vi "WS1050 36 DUT CV Curve Ver1.1.vi"() -> ()   [LabVIEW 2012]
uses:
  All Driver/Keithley/2012_Keithley 24XX/Keithley 24XX.lvlib
  WS_VCAP Driver 029/Source/WSVCAP Shell/Type Defs/WSVCAP SHL I2C DUT Mask Mode Enum.ctl
panel:
  out "VISA resource name out":refnum<visa-resource-name>="GPIB0::3::INSTR"
  out "error out 2":errorcluster={"status"=TRUE, "code"=-63192, "source"="niLvFpga_Open_PXI-7813R.vi"}
  in  "Reg1_Bit Cntrl":string[](array[string])=["01", "02", "04", "08", "10", "20", "40", "80", "03", "06", "0C", "D8", "33", "66", "CC", "07", "0E", "1C", "38", "70", "E0", "0F", "1E", "3C", "78", "F0", "1F", "3E", "7C", "F8", "3F", "7E", "FC", "7F", "FE", "FD", "FB", "F7", "EF", "DF", "BF", "7F", "FC", "F9", "F3", "E7", "CF", "9F", "3F", "F8", "F1", "E3", "C7", "8F", "1F", "F0", "E1", "C3", "87", "0F", "E0", "C1", "83", "07", "C0", "81", "03", "AA", "55", "00"]
  out "date string":string="5/19/2014"
  out "PS1 Out":refnum<visa-resource-name>
  out "Ke2000 Out":refnum<visa-resource-name>="GPIB0::9::INSTR"
  in  "Tab Control":T1(tab)
  in  "Board#":string="BRD5"
  in  "Serial Number":string[][](table)=[["DUT", "SN"], ["DUT1", "1"], ["DUT2", "2"], ["DUT3", "3"], ["DUT4", "4"], ["DUT5", "5"], ["DUT6", "6"], ["DUT7", "7"], ["DUT8", "8"], ["DUT9", "9"], ["DUT10", "10"], ["DUT11", "11"], ["DUT12", "12"], ["DUT13", "13"], ["DUT14", "14"], ["DUT15", "15"], ["DUT16", "16"], ["DUT17", "17"], ["DUT18", "18"], ["DUT19", "19"], ["DUT20", "20"], ["DUT21", "21"], ["DUT22", "22"], ["DUT23", "23"], ["DUT24", "24"], ["DUT25", "25"], ["DUT26", "26"], ["DUT27", "27"], ["DUT28", "28"], ["DUT29", "29"], ["DUT30", "30"], ["DUT31", "31"], ["DUT32", "32"], ["DUT33", "33"], ["DUT34", "34"], ["DUT35", "35"], ["DUT36", "36"]]
  in  "Wafer#":string="T7-EB"
  in  "File Name":string="CYC_WS1050_T7_EB_65C_40V_25DC_EMPTY_BRD5_141017_1"
  in  "TMN DC\\CAP Data Log File Path":path=path "C:/WS1050 36 DUT Data"
  in  "Test Program":string="WS1050 36 DUT CV Curve Ver1.1"
  out "Current Date":string="8/28/2014"
  out "Current Time":string="0950"
  in  "Start Date":string="10/21/2014"
  in  "Start Time":string="1542"
  in  "Comment":string="CYC65C40V"
  in  "OK Button":bool
  in  "Calibration":bool
  in  "Verify CP":bool
  in  "CP Setting":i32(ring) items=["CP OFF", "CP ON", "CP 35V", "CP 40V", "DVA ON", "DVA OFF", "REG1 ON", "REG1 OFF", "REG2 ON", "REG2 OFF", "REG3 ON", "REG3 OFF"]
  in  "Stop Calibration":bool
  in  "Set VDD":dbl=3.3 format="%.3g"
  in  "Clock Rate (Hz)":dbl=1000000.0 caption="Meas Speed" format="%.1p Hz"
  out "AR  Measurent(Hz)":dbl
  in  "PS1 Source":refnum<visa-resource-name>="GPIB0::5::INSTR"
  in  "Ke2000":refnum<visa-resource-name>="GPIB0::9::INSTR"
  in  "CP to HD/Cycle":i32(ring)=1 items=["CP HDC 35V", "CP HDC 40.25V", "CP HDC 27.5V", "CP HDC 30.5V", "CP HDC 44V"]
  out "Simulate FPGA":bool
  out "Online":bool
  in  "Ke2400":refnum<visa-resource-name>="GPIB0::3::INSTR"
  in  "Initialize AD7747":bool
  in  "DUT Mask Mode":T2=enum."All"
  in  "RFFE Slave Address":u8=7 caption="Slave Address" format="0x%02x"
  out "Activity Log":string="05/19/2014 -- 12:24:35.853::WSVCAP::APP::Application Started\n05/19/2014 -- 12:24:37.606::WSVCAP::WSVCAP SHL::WR I2C-REG:0x0A;MASK:0xFFFFFFFFFFFF;C1 DATA:22:22:22:22:22:22:22:22:22:22:22:22:22:22:22:22;C2 DATA:22:22:22:22:22:22:22:22:22:22:22:22:22:22:22:22;C3 DATA:22:22:22:22:22:22:22:22:22:22:22:22:22:22:22:22\r\n05/19/2014 -- 12:24:37.773::WSVCAP::WSVCAP SHL::WR I2C-ST:0,0,4,1\r\n05/19/2014 -- 12:24:37.903::WSVCAP::WSVCAP SHL::RD I2C-BYTES:4;ADD:0x00;MASK:0xFFFFFFFFFFFF\r\n05/19/2014 -- 12:24:38.045::WSVCAP::WSVCAP SHL::RD I2C:C1 DATA:2:2:2:2:2:2:2:2:2:2:2:2:2:2:2:2|A7:A9:AA:82:82:7F:82:81:82:81:83:82:81:82:82:81|46:36:BB:88:44:A3:E9:2B:32:20:ED:25:BB:3D:68:B|2C:6A:EB:A7:22:56:FE:CC:36:82:D7:B0:3B:48:F9:CC;C2 DATA:2:2:2:2:2:2:2:2:2:2:2:2:2:2:2:2|94:94:94:80:80:80:80:80:81:7E:7E:81:80:7E:80:80|47:33:15:82:62:B:E8:1C:D7:C3:7D:41:7C:B7:4C:2A|C4:B4:AE:8:1E:D1:4E:37:11:C0:6F:63:42:9D:63:B5;C3 DATA:2:2:2:2:2:2:2:2:2:2:2:2:2:2:2:2|95:95:95:81:81:7E:81:80:84:7D:80:83:81:7E:7F:80|AB:C4:14:B5:7B:52:DF:C9:79:5D:5F:30:99:31:1E:F4|6E:5C:F7:A8:C3:EB:7B:EF:33:92:89:77:4D:67:75:DD;STATUS:0:0:4:0\r\n05/19/2014 -- 12:24:38.046::WSVCAP::WSVCAP SHL::WR I2C-REG:0x0A;MASK:0xFFFFFFFFFFFF;C1 DATA:22:22:22:22:22:22:22:22:22:22:22:22:22:22:22:22;C2 DATA:22:22:22:22:22:22:22:22:22:22:22:22:22:22:22:22;C3 DATA:22:22:22:22:22:22:22:22:22:22:22:22:22:22:22:22\r\n05/19/2014 -- 12:24:38.089::WSVCAP::WSVCAP SHL::WR I2C-ST:0,0,4,1\r\n05/19/2014 -- 12:24:38.219::WSVCAP::WSVCAP SHL::RD I2C-BYTES:4;ADD:0x00;MASK:0xFFFFFFFFFFFF\r\n05/19/2014 -- 12:24:38.362::WSVCAP::WSVCAP SHL::RD I2C:C1 DATA:2:2:2:2:2:2:2:2:2:2:2:2:2:2:2:2|A7:AB:AA:82:82:82:83:83:82:82:82:82:7F:82:82:81|4B:32:96:83:3E:61:43:17:25:62:AB:4D:A2:40:2E:5|3C:76:2B:B4:EE:E4:A9:1A:AA:A:26:C7:21:2E:87:5B;C2 DATA:2:2:2:2:2:2:2:2:2:2:2:2:2:2:2:2|94:94:94:80:80:80:80:80:80:7F:80:81:80:80:7F:80|4A:32:19:7D:19:6C:79:46:61:7F:4B:B8:A5:30:F3:14|B4:70:A:8C:9C:DC:43:FA:1E:A:C6:21:A:A9:13:F3;C3 DATA:2:2:2:2:2:2:2:2:2:2:2:2:2:2:2:2|95:97:94:81:80:81:82:81:80:7E:81:84:7F:81:80:80|B2:32:D0:A7:9E:4C:AB:D4:EE:D9:F0:82:B7:91:7:FF|C1:91:B6:3D:D8:E:1B:4F:9F:6A:F1:6C:E7:3F:7:BA;STATUS:0:0:4:0\r\n05/19/2014 -- 12:24:38.364::WSVCAP::WSVCAP SHL::WR I2C-REG:0x0A;MASK:0xFFFFFFFFFFFF;C1 DATA:22:22:22:22:22:22:22:22:22:22:22:22:22:22:22:22;C2 DATA:22:22:22:22:22:22:22:22:22:22:22:22:22:22:22:22;C3 DATA:22:22:22:22:22:22:22:22:22:22:22:22:22:22:22:22\r\n05/19/2014 -- 12:24:38.406::WSVCAP::WSVCAP SHL::WR I2C-ST:0,0,4,1\r\n05/19/2014 -- 12:24:38.536::WSVCAP::WSVCAP SHL::RD I2C-BYTES:4;ADD:0x00;MASK:0xFFFFFFFFFFFF\r\n05/19/2014 -- 12:24:38.678::WSVCAP::WSVCAP SHL::RD I2C:C1 DATA:2:2:2:2:2:2:2:2:2:2:2:2:2:2:2:2|A7:A9:AB:82:82:81:82:82:82:82:82:82:82:82:82:81|46:71:4C:87:43:3D:7F:FC:25:4F:8E:54:97:3E:60:8C|AA:F4:1F:B5:CE:43:1F:36:9:87:9C:78:86:5:B6:8E;C2 DATA:2:2:2:2:2:2:2:2:2:2:2:2:2:2:2:2|94:94:94:80:7F:7F:80:80:80:80:80:81:80:80:80:80|49:36:18:7D:6E:C5:E4:3C:81:2E:41:D3:75:71:E3:72|E8:D3:E6:D1:E0:48:AE:D4:54:D:E8:8E:B4:41:68:4;C3 DATA:2:2:2:2:2:2:2:2:2:2:2:2:2:2:2:2|95:95:95:81:7F:7F:81:81:81:81:81:84:81:81:82:81|B3:F5:90:AB:82:69:7B:93:D0:77:E8:D5:E8:8C:84:E8|B9:AC:EE:2B:B6:71:8F:4A:74:31:56:BB:8A:B7:A0:C8;STATUS:0:0:4:0\r\n05/19/2014 -- 12:24:38.681::WSVCAP::WSVCAP SHL::WR I2C-REG:0x0A;MASK:0xFFFFFFFFFFFF;C1 DATA:22:22:22:22:22:22:22:22:22:22:22:22:22:22:22:22;C2 DATA:22:22:22:22:22:22:22:22:22:22:22:22:22:22:22:22;C3 DATA:22:22:22:22:22:22:22:22:22:22:22:22:22:22:22:22\r\n05/19/2014 -- 12:24:38.723::WSVCAP::WSVCAP SHL::WR I2C-ST:0,0,4,1\r\n05/19/2014 -- 12:24:38.854::WSVCAP::WSVCAP SHL::RD I2C-BYTES:4;ADD:0x00;MASK:0xFFFFFFFFFFFF\r\n05/19/2014 -- 12:24:38.996::WSVCAP::WSVCAP SHL::RD I2C:C1 DATA:2:2:2:2:2:2:2:2:2:2:2:2:2:2:2:2|A7:A9:AA:82:82:7F:83:81:82:81:84:82:7F:82:7F:82|43:FB:E:7F:3C:AD:35:35:26:A2:6C:21:4B:3D:8:6|63:9A:E1:F3:95:32:91:42:90:3C:78:1F:5C:D7:5F:D8;C2 DATA:2:2:2:2:2:2:2:2:2:2:2:2:2:2:2:2|94:94:94:80:80:80:80:80:81:80:7E:81:80:7E:7F:80|48:36:18:7F:5E:3D:69:83:DE:AE:A1:9E:31:AE:BB:96|15:A0:44:17:13:FD:CC:C8:6D:B2:EF:A7:C:C7:3B:F;C3 DATA:2:2:2:2:2:2:2:2:2:2:2:2:2:2:2:2|95:96:94:81:81:7E:82:80:84:80:80:84:7F:7E:7D:82|AD:3B:6D:A9:7C:57:9D:F5:7A:96:23:5C:36:2D:ED:5A|CD:46:DB:3B:C7:BD:70:60:33:B8:B:F7:63:A:51:4D;STATUS:0:0:4:0\r\n05/19/2014 -- 12:24:38.998::WSVCAP::WSVCAP SHL::WR I2C-REG:0x0A;MASK:0xFFFFFFFFFFFF;C1 DATA:22:22:22:22:22:22:22:22:22:22:22:22:22:22:22:22;C2 DATA:22:22:22:22:22:22:22:22:22:22:22:22:22:22:22:22;C3 DATA:22:22:22:22:22:22:22:22:22:22:22:22:22:22:22:22\r\n05/19/2014 -- 12:24:39.040::WSVCAP::WSVCAP SHL::WR I2C-ST:0,0,4,1\r\n05/19/2014 -- 12:24:39.170::WSVCAP::WSVCAP SHL::RD I2C-BYTES:4;ADD:0x00;MASK:0xFFFFFFFFFFFF\r\n05/19/2014 -- 12:24:39.311::WSVCAP::WSVCAP SHL::RD I2C:C1 DATA:2:2:2:2:2:2:2:2:2:2:2:2:2:2:2:2|A7:AA:AB:82:82:81:82:81:82:81:82:82:82:82:7F:82|44:F1:90:87:45:44:C8:2C:2C:F1:FC:1B:94:3B:3C:75|4A:49:95:19:99:73:64:3:23:24:F3:A2:5E:7F:C4:B6;C2 DATA:2:2:2:2:2:2:2:2:2:2:2:2:2:2:2:2|94:94:94:80:80:80:80:7F:80:80:7E:80:80:7E:7F:80|4C:36:17:7D:A8:9F:DE:C7:53:6D:8A:F4:41:A5:C6:E0|90:2E:24:C:D9:22:E4:76:3B:40:1D:53:33:B1:3E:4D;C3 DATA:2:2:2:2:2:2:2:2:2:2:2:2:2:2:2:2|95:97:95:81:81:7F:81:80:80:81:7F:82:81:7E:7D:82|AE:2B:A7:AB:CC:CD:A4:38:FD:17:80:F2:92:2D:45:C4|76:E5:D:B9:AD:B5:BA:8D:28:32:9E:42:B7:20:4A:D9;STATUS:0:0:4:0\r\n05/19/2014 -- 12:24:39.313::WSVCAP::WSVCAP SHL::WR I2C-REG:0x0A;MASK:0xFFFFFFFFFFFF;C1 DATA:22:22:22:22:22:22:22:22:22:22:22:22:22:22:22:22;C2 DATA:22:22:22:22:22:22:22:22:22:22:22:22:22:22:22:22;C3 DATA:22:22:22:22:22:22:22:22:22:22:22:22:22:22:22:22\r\n05/19/2014 -- 12:24:39.355::WSVCAP::WSVCAP SHL::WR I2C-ST:0,0,4,1\r\n05/19/2014 -- 12:24:39.486::WSVCAP::WSVCAP SHL::RD I2C-BYTES:4;ADD:0x00;MASK:0xFFFFFFFFFFFF\r\n05/19/2014 -- 12:24:39.628::WSVCAP::WSVCAP SHL::RD I2C:C1 DATA:2:2:2:2:2:2:2:2:2:2:2:2:2:2:2:2|A7:A9:AA:82:82:82:83:82:82:82:82:82:7F:82:7F:82|47:18:E4:87:3E:E7:6:65:25:92:37:38:A8:3E:89:85|7C:A7:7:2B:A3:7A:EC:EF:89:ED:F4:D3:D8:BC:3A:F5;C2 DATA:2:2:2:2:2:2:2:2:2:2:2:2:2:2:2:2|94:94:94:80:7F:80:80:7F:81:80:7E:80:80:80:81:80|49:37:17:80:76:25:6A:F8:DF:55:97:4D:B8:5B:2B:B1|13:E3:9A:3E:1A:2D:4F:B6:DB:E9:61:FA:8B:D6:9:CC;C3 DATA:2:2:2:2:2:2:2:2:2:2:2:2:2:2:2:2|95:95:95:81:7F:80:82:81:84:80:7F:81:80:81:7F:82|AF:93:3B:AF:5B:11:82:E4:7E:C3:2D:72:9:96:D9:A|DB:96:F2:10:5F:64:9A:C6:98:12:27:7D:10:D3:20:D9;STATUS:0:0:4:0\r\n05/19/2014 -- 12:24:40.132::WSVCAP::WSVCAP SHL::CLOSE\r\n"
  in  "C1 Cap DAC":u8=128 caption="B Data In" format="0x%02x"
  in  "C2 Cap DAC":u8=128 caption="B Data In" format="0x%02x"
  in  "C3 Cap DAC":u8=128 caption="B Data In" format="0x%02x"
  out "IDD Brd(uA)":string
  in  "Control Panel":T3={"Verify Socket"=FALSE, "HD/CYC"=FALSE, "E-CAL"=FALSE, "DVA"=FALSE, "VPI"=TRUE, "VSA"=FALSE, "HS"=FALSE}
  out "Verify Socket":bool
  out "HD/CYC":bool
  out "E-CAL":bool
  out "DVA":bool
  out "VPI":bool
  out "VSA":bool
  out "HS":bool
  in  "Lot#":string="WS1050"
  out "AD7747 Values":string[][](table)
  in  "Freq(Hz)":string="NA"
  in  "Reset P/S":bool
  in  "Test Sequences":i32(ring) items=["C1_C2_C3", "C2_C1_C3", "C3_C2_C1"]
  in  "WS1050/51":bool=TRUE
  in  "CP with DVA ON":i32(ring) items=["CP HDC 35V", "CP HDC 40.25V", "CP HDC 27.5V", "CP HDC 30.5V", "CP HDC 44V"]
  in  "CP Sweep":bool=TRUE
  in  "Serialize":bool
  in  "Start No":i32=1
  in  "VPI Name":string[](array[string])=["All Drivers ON"]
  in  "VPI_Cmd":string[](array[string])=["3B"]
  in  "Temperature":string="25C"
  out "40V_1":string[][](table)
  out "NOM IDD OFF(uA)":string
  out "40V_2":string[][](table)
  out "40V_3":string[][](table)
  out "Previous Time":string="12:20:26 PM"
  out "STATUS":string="Idle...."
  out "Total Delta C2(pF)":string[](array[string])
  out "Total Delta C1(pF)":string[](array[string])
  out "Total Delta C3(pF)":string[](array[string])
  out "RB Reg for HD/Cycle":string[](array[string])
  out "VPI C2":string[][](table)
  out "VPI C3":string[][](table)
  out "NOM IDD ON (uA)":string
  out "IDD_HD/CYC (uA)":string="164.601255E+0"
  in  "stop":bool
  out "IDD Stdby(uA)":string="2.606990E+0"
  out "VPI C1":string[][](table)
  in  "TTF Completed":i32=60
  out "Loop Completed":i32
  out "VSA_V1":string[][](table)
  out "VSA_V2":string[][](table)
  out "VSA_V3":string[][](table)
  in  "VSA Voltage(V)":dbl[](array[numeric])=[-27.0, 0.0, 27.0]
  in  "X Repeat":i32=100
  out "% Delta C_T0":string[][](array[string])
  out "% Delta C":string[][](array[string])
  out "EFuse RB T0":string[](array[string])
  out "Current EFuse Read back":string[](array[string])
  out "EFuse Readback Status":bool[](array[boolean])
  in  "DeltaC Target Setting(pF)":dbl=7.375
  out "error out":errorcluster
  in  "error in (no error)":errorcluster
  in  "Bank 2":i32(ring)=1 items=["C1", "C2", "C3", "D_C1", "D_C2", "D_C3"]
  out "DeltaC Change_1":dbl[][](graph) caption="(Y) Multi Plot 2"
  out "DeltaC Change_2":dbl[][](graph) caption="(Y) Multi Plot 2"
  out "DeltaC Change_3":dbl[][](graph) caption="(Y) Multi Plot 2"
  in  "Debug":bool
  in  "No of Rows\nFrom Spread Sheet":i32
  in  "Plot Delta Cmin":bool=TRUE
  in  "Plot":T4(ring)
  in  "Bank 1":i32(ring) items=["C1", "C2", "C3", "D_C1", "D_C2", "D_C3"]
  in  "Bank 3":i32(ring)=2 items=["C1", "C2", "C3", "D_C1", "D_C2", "D_C3"]
  in  "Col C1":i32=5
  in  "Col C2":i32=6
  in  "Col C3":i32=7
  # "Company:  WiSpry Inc\n20 Fairbanks Ste 198 Irvine CA 92618\n\nAuthor:  Andy V Tran\nCreated:  01/07/2015\nLabVIEW 2012 Pro\nTest Program:  WS1050 36 DUT CV Curve ver1.0\nFPGA: WS_VCAP Driver 029"
  # "Note for HD Duty Cycle:\n\n1.  Set HD/Cycle to Completed = 4320 minutes = 72 hours \n(T0 24hrs HD, T2 48hrs HD_Duty Cycle);  Default Setting\n2.  Set Time to Start HD Duty Cycle = 1440 = 24 hours\n3.  Set Time All ON = 120s = 2 minutes\n4.  Set Time All OFF = 120s = 2 minutes\n5.  No of Loops to RP = 3600s/(Time ALL ON(s) + Time ALL + OFF(s))\n6.  X Repeat = X runs\n7.  Set TTF Completed = Repeat X item1 to Stop.\n8.  Stop Test, set TTF Completed = Total Time Completed."
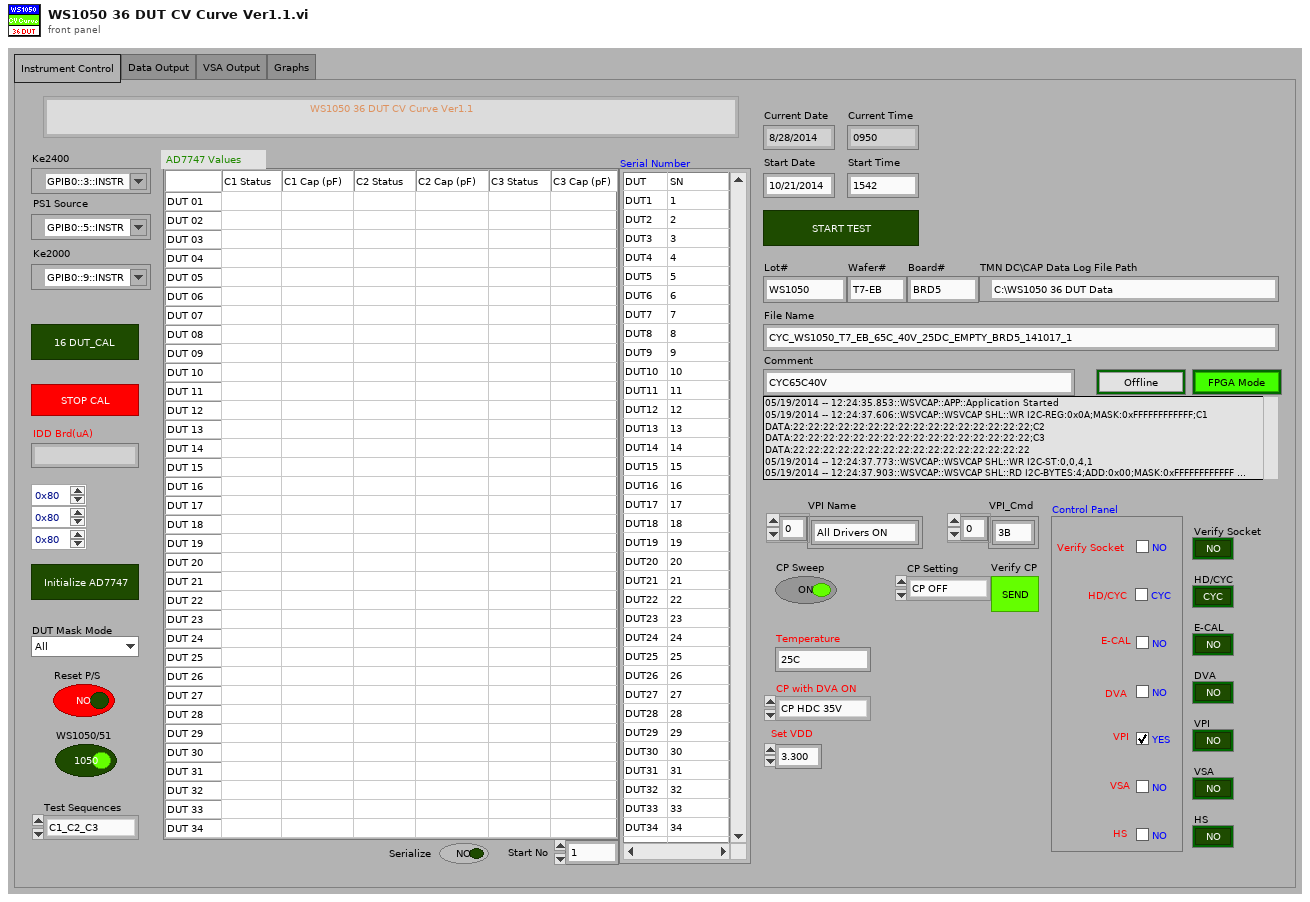
[diagram p1: front panel]
types:
  T1 = enum32{"Instrument Control", "Data Output", "VSA Output", "Graphs"}
  T2 = typedef "WSVCAP SHL I2C DUT Mask Mode Enum.ctl" = enum16{"Custom", "C1", "C2", "C3", "All"}
  T3 = cluster{"Verify Socket":bool, "HD/CYC":bool, "E-CAL":bool, "DVA":bool, "VPI":bool, "VSA":bool, "HS":bool}
  T4 = enum16{"ALL DUTs", "DUT 01", "DUT 02", "DUT 03", "DUT 04", "DUT 05", "DUT 06", "DUT 07", "DUT 08", "DUT 09", "DUT 10", "DUT 11", "DUT 12", "DUT 13", "DUT 14", "DUT 15", "DUT 16", "DUT 17", "DUT 18", "DUT 19", "DUT 20", "DUT 21", "DUT 22", "DUT 23", "DUT 24", "DUT 25", "DUT 26", "DUT 27", "DUT 28", "DUT 29", "DUT 30", "DUT 31", "DUT 32", "DUT 33", "DUT 34", "DUT 35", "DUT 36"}
  T5 = typedef "WSVCAP SHL Core System Cluster.ctl" = cluster{"Settings":T6, "FPGA Resource":tag, "Online":bool, "I2C Wait Ticks":u32, "SPI Wait Ticks":u32, "RFFE Wait Ticks":u32}
  T6 = typedef "WSVCAP SHL I2C Settings Cluster.ctl" = cluster{"FPGA Resource Name":string, "I2C Slave Address":u8, "I2C Clock Rate (Hz)":dbl, "SPI Clock Rate (Hz)":dbl, "RFFE Slave Address":u8, "RFFE Clock Rate (Hz)":dbl, "Simulate FPGA":bool, "C1 Cap DAC Default":u8, "C2 Cap DAC Default":u8, "C3 Cap DAC Default":u8}
  T7 = enum16{"Idle...", "Voltage 1", "Voltage 2", "Voltage 3"}[]
  T8 = cluster{"Test Program ":string, "Comment":string, "Data Out":string, "Data Out":string, "Data Out":string, string, "Data Out":string, "Data Out":string, "Data Out":string, "Freq(Hz)":string, "Board#":string}
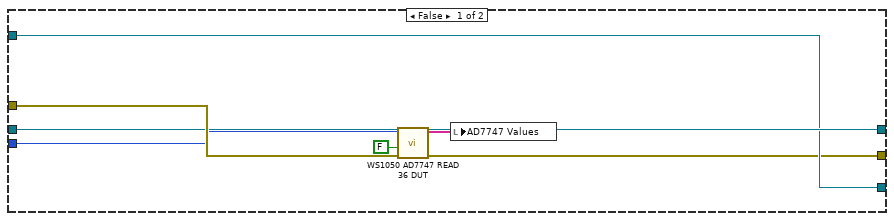
[diagram p9: hidden frame]
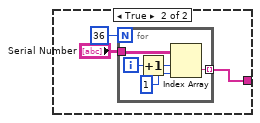
[diagram p10: hidden frame]
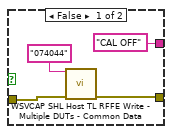
[diagram p11: hidden frame]
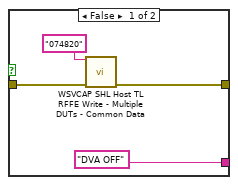
[diagram p12: hidden frame]
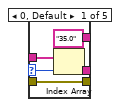
[diagram p13: hidden frame]
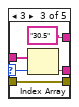
[diagram p14: hidden frame]
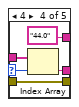
[diagram p15: hidden frame]
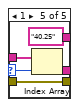
[diagram p16: hidden frame]
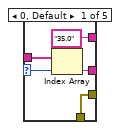
[diagram p17: hidden frame]
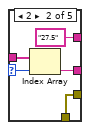
[diagram p18: hidden frame]
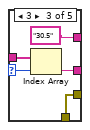
[diagram p19: hidden frame]
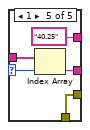
[diagram p20: hidden frame]
diagram:
  w18 = TRUE
  w24 = u16 0 items=["Off", "Moving Filter", "Repeating Filter"] ("Digital Filter (0: Off)")
  w25 = u16 7 items=["3.5 Digits"=4, "4.5 Digits"=5, "5.5 Digits"=6, "6.5 Digits"=7] ("Resolution (7: 6.5 digits)")
  n1 = case shown="True" w18 {
    tunnel: "error in (no error)" -> [w31 w32]
    tunnel: [w31 w39] -> w5
    frame False {
    }
    frame True {
      n2 = call "WSVCAP SHL Host TL Initialize.vi"("error in"=w32) -> ("error out"=w33:errorcluster)  [unwired: 13 in, 1 out]
      n3 = control-ref of="Activity Log"() -> (w35:refnum<vi>)
      n4 = call "ACT LG Activity Log Core.vi"("Display Ref"=w35, "Source"="WSVCAP", "Error In (no error)"=w33) -> ("Error Out"=w34:errorcluster)  [unwired: 11 in, 1 out]
      n5 = call "WSVCAP SHL Host TL Status Manager.vi"("error in"=w34) -> ("System Out"=w40:T5, "error out"=w39:errorcluster)  [unwired: 13 in]
      n6 = Unbundle By Name(w40) -> ("Online"=→"Online":bool, "Settings.Simulate FPGA"=→"Simulate FPGA":bool)
    }
  }
  n7 = case shown="True" TRUE {
    tunnel: w5 -> [w41 w46]
    tunnel: [w42 w45] -> w15
    tunnel: [w41 w44] -> w9
    tunnel: "Ke2400" -> [w42 w43]
    frame False {
    }
    frame True {
      n8 = VISA Write(VISA resource name=w43, write buffer="SOUR:FUNC VOLT;VOLT:MODE FIX;RANG 100;LEV 0.0;:SENS:FUNC \"CURR\";CURR:PROT 60E-3;RANG 100E-3;:OUTP ON", error in (no error)=w46) -> (VISA resource name out=w45:refnum<visa-resource-name>, error out=w44:errorcluster)  [unwired: 1 out]
    }
  }
  n9 = case shown="True" "Reset P/S" {
    tunnel: "PS1 Source" -> [w48 w55]
    tunnel: [w48 w53] -> w29
    tunnel: w5 -> [w49 w51]
    tunnel: [w49 w50] -> w4
    frame False {
    }
    frame True {
      n10 = call "Agilent 3631A Initialize.vi"("error in (no error)"=w51, "Default"=FALSE ("Reset? (T: Yes)"), "Reset"=TRUE ("ID Query? (T: Yes)"), "VISA resource name"=w55) -> ("error out"=w50:errorcluster, "VISA resource name out"=w53:refnum<visa-resource-name>)  [unwired: 6 in]
    }
  }
  n11 = call "Ke2000 Initialize.vi"("error in (no error)"=w5, "VISA resource name"="Ke2000") -> ("error out"=w26:errorcluster, "VISA resource name out"=w27:refnum<visa-resource-name>)  [unwired: 8 in]
  n12 = call "Ke2000 Configure DC Current.vi"("Resolution (7: 6.5 digits)"=w25, "Digital Filter (0: Off)"=w24, "Auto Range? (T: Auto)"=FALSE, "error in"=w26, "Custom Range (0 A)"=1.0, "VISA resource name"=w27) -> ("error out"=w6:errorcluster, "VISA resource name out"=w22:refnum<visa-resource-name>)  [unwired: 4 in]
  n13 = Merge Errors(w9, w6, w4) -> (w16:errorcluster)
  n14 = while {
    tunnel: w16 -> [w61]
    tunnel: [w64] -> w12
    tunnel: w29 -> [w68]
    tunnel: w22 -> [w69]
    tunnel: [w78] -> w21
    tunnel: [w77] -> w20
    tunnel: w15 -> [w75]
    tunnel: [w74] -> w13
    tunnel: [FALSE ("stop")] -> w7
    i -> [w76]
    stop <- w80 stop-if-true
    n15 = case shown="0" w76 {
      tunnel: w61 -> [w91 w92]
      tunnel: [w90 w92] -> w71
      tunnel: "RFFE Slave Address" -> [w88 _]
      frame 0 {
        w84 = dbl[][] []
        w83 = "" ("uA")
        w85 = string[][] []
        w86 = string[] [] ("EFuse Read back")
        n16 = local write "RB Reg for HD/Cycle"(w86) -> ()
        n17 = local write "Current EFuse Read back"(w86) -> ()
        n18 = local write "EFuse RB T0"(w86) -> ()
        n19 = local write "Total Delta C1(pF)"(w86) -> ()
        n20 = local write "Total Delta C2(pF)"(w86) -> ()
        n21 = local write "Total Delta C3(pF)"(w86) -> ()
        n22 = local write "VPI C2"(w85) -> ()
        n23 = local write "VSA_V3"(w85) -> ()
        n24 = local write "VSA_V1"(w85) -> ()
        n25 = local write "40V_2"(w85) -> ()
        n26 = local write "40V_1"(w85) -> ()
        n27 = local write "NOM IDD OFF(uA)"(w83) -> ()
        n28 = local write "NOM IDD ON (uA)"(w83) -> ()
        n29 = local write "IDD Brd(uA)"(w83) -> ()
        n30 = local write "VSA_V2"(w85) -> ()
        n31 = local write "VPI C1"(w85) -> ()
        n32 = local write "VPI C3"(w85) -> ()
        n33 = local write "% Delta C"(w85) -> ()
        n34 = local write "% Delta C_T0"(w85) -> ()
        n35 = local write "40V_3"(w85) -> ()
        n36 = call "WSVCAP SHL Host TL RFFE Configure.vi"("RFFE Slave Address"=w88, "Clock Rate (Hz)"="Clock Rate (Hz)", "error in"=w91) -> ("Actual Rate (Hz)"=→"AR  Measurent(Hz)":dbl, "error out"=w90:errorcluster)  [unwired: 11 in]
        n37 = local write "DeltaC Change_3"(w84) -> ()
        n38 = local write "DeltaC Change_1"(w84) -> ()
        n39 = local write "DeltaC Change_2"(w84) -> ()
      }
      frame 1, Default {
      }
    }
    n40 = while {
      tunnel: ["stop"] -> w73
      tunnel: w71 -> [w113]
      tunnel: [w105] -> w65
      tunnel: w68 -> [w112]
      tunnel: w69 -> [w107]
      tunnel: [w108] -> w67
      tunnel: [w106] -> w66
      tunnel: [w103] -> w63
      tunnel: [w102] -> w62
      tunnel: [w101] -> w60
      tunnel: [w100] -> w59
      tunnel: [w99] -> w58
      tunnel: [w98] -> w57
      tunnel: [w97] -> w56
      stop <- w120 stop-if-true
      # "Set Date & Time to Start Test"
      n41 = case shown="True" "Initialize AD7747" {
        tunnel: w113 -> [w129 w134]
        tunnel: [w129 w130] -> w96
        tunnel: w112 -> [w128 w132]
        tunnel: [w128 w131] -> w111
        frame False {
        }
        frame True {
          w135 = T7 [enum."Voltage 2", enum."Voltage 3", enum."Voltage 1"] items=["Idle...", "Voltage 1", "Voltage 2", "Voltage 3"]
          n42 = for {
            tunnel: w132 -> [w145]
            tunnel: w135 -> [w143] mode=indexing
            tunnel: [w142] -> w131
            shift-right: [w138] -> w133
            shift-left: w134 -> [w146]
            n43 = local read "Set VDD"() -> (w141:dbl)
            n44 = call "E3631A_Voltage Controller.vi"("VISA resource name"=w145, "I_VDD(A)"=0.5, "Channel Controller"=w143, "Voltage 1"=w141, "Voltage 2"=3.3, "error in (no error)"=w146, "I_3.3V (A)"=0.5) -> ("VISA resource name out"=w142:refnum<visa-resource-name>, "error out"=w137:errorcluster)  [unwired: 7 in]
            n45 = call "Delay T4.vi"("milliseconds to wait"=u32 100, "error in (no error)"=w137) -> ("error out"=w138:errorcluster)  [unwired: 9 in]
          }
          n46 = call "WS1050_AD7747_Init 36DUT.vi"("error in"=w133) -> ("error out"=w130:errorcluster)  [unwired: 10 in]
        }
      }
      n47 = call "Time_stamp.vi"() -> ("date/time string"=w125:string, "date string"=w127:string)  [unwired: 2 in]
      "Current Date" <- w127
      "Current Time" <- w125
      n48 = Equal?(x=w127, y="Start Date") -> (x = y?=w123:bool)
      n49 = Equal?(x=w125, y="Start Time") -> (x = y?=w122:bool)
      n50 = And(x=w123, y=w122) -> (x .and. y?=w119:bool)
      n51 = Compound Arithmetic op=OR(w119, "OK Button", "stop") -> (w120:bool)
      n52 = case shown="True" "Calibration" {
        tunnel: w96 -> [w176 w193]
        tunnel: [w170 w190] -> w94
        tunnel: w111 -> [w175 w189]
        tunnel: "DUT Mask Mode" -> [w174 w185]
        tunnel: [w175 w184] -> w109
        tunnel: w107 -> [w173 w180]
        tunnel: [w173 w177] -> w106
        frame False {
          n53 = call "WS1050 AD7747 READ 36 DUT.vi"("error in"=w176, "Log (T)"=FALSE, "DUT Mask Mode (All)"=w174) -> ("error out"=w170:errorcluster, "AD7747 Values"=w171:string[][])  [unwired: 7 in]
          n54 = local write "AD7747 Values"(w171) -> ()
        }
        frame True {
          n55 = flat-sequence {
            tunnel: w193 -> [w202]
            tunnel: [w197] -> w192
            tunnel: w189 -> [w201]
            tunnel: [w200] -> w188
            tunnel: w185 -> [w199]
            tunnel: [w199] -> w186
            tunnel: w180 -> [w195]
            tunnel: [w194] -> w179
            tunnel: w192 -> [w226]
            tunnel: [w225] -> w191
            tunnel: w188 -> [w224]
            tunnel: [w224] -> w187
            tunnel: w186 -> [w223]
            tunnel: "C1 Cap DAC" -> [w219]
            tunnel: "C2 Cap DAC" -> [w218]
            tunnel: "C3 Cap DAC" -> [w217]
            tunnel: w179 -> [w216]
            tunnel: [w216] -> w178
            tunnel: w191 -> [w235]
            tunnel: [w238] -> w190
            tunnel: w187 -> [w237]
            tunnel: [w234] -> w184
            tunnel: w178 -> [w233]
            tunnel: [w233] -> w177
            frame #0 {
              w203 = T7 [enum."Voltage 2", enum."Voltage 3", enum."Voltage 1"] items=["Idle...", "Voltage 1", "Voltage 2", "Voltage 3"]
              n56 = for {
                tunnel: w201 -> [w214]
                tunnel: w203 -> [w212] mode=indexing
                tunnel: [w211] -> w200
                shift-right: [w209] -> w196
                shift-left: w202 -> [w215]
                n57 = local read "Set VDD"() -> (w206:dbl)
                n58 = call "E3631A_Voltage Controller.vi"("VISA resource name"=w214, "I_VDD(A)"=0.5, "Channel Controller"=w212, "Voltage 1"=w206, "Voltage 2"=3.3, "error in (no error)"=w215, "I_3.3V (A)"=0.5) -> ("VISA resource name out"=w211:refnum<visa-resource-name>, "error out"=w208:errorcluster)  [unwired: 7 in]
                n59 = call "Delay T4.vi"("milliseconds to wait"=u32 100, "error in (no error)"=w208) -> ("error out"=w209:errorcluster)  [unwired: 9 in]
              }
              n60 = call "Ke2000 Single Reading.vi"("error in (no error)"=w196, "VISA resource name"=w195) -> ("error out"=w197:errorcluster, "VISA resource name out"=w194:refnum<visa-resource-name>, "uA"=→"IDD Brd(uA)":string)  [unwired: 5 in, 2 out]
              n61 = One Button Dialog(message="Please verify all sockets should be empty...") -> ()  [unwired: 1 in, 1 out]
            }
            frame #1 {
              n62 = call "WS1050 CAPDAC Setting.vi"("DUT Mask Mode (All)"=w223, "error in"=w226, "C3 Cap DAC"=w217, "C2 Cap DAC"=w218, "C1 Cap DAC"=w219) -> ("error out"=w221:errorcluster)  [unwired: 6 in]
              n63 = call "WS1050 OFFSET CAL.vi"("error in"=w221, "OFFSET CAL"=TRUE ("Read?")) -> ("error out"=w220:errorcluster)  [unwired: 9 in]
              n64 = while {
                tunnel: w220 -> [w232]
                tunnel: [w231] -> w225
                tunnel: w223 -> [w229]
                stop <- "Stop Calibration" stop-if-true
                n65 = call "WS1050 AD7747 READ 36 DUT.vi"("error in"=w232, "Log (T)"=FALSE, "DUT Mask Mode (All)"=w229) -> ("error out"=w231:errorcluster, "AD7747 Values"=→"AD7747 Values":string[][])  [unwired: 7 in]
              }
            }
            frame #2 {
              w236 = T7 [enum."Voltage 2", enum."Voltage 3", enum."Voltage 1"] items=["Idle...", "Voltage 1", "Voltage 2", "Voltage 3"]
              n66 = for {
                tunnel: w237 -> [w250]
                tunnel: w236 -> [w247] mode=indexing
                tunnel: [w246] -> w234
                shift-right: [w242] -> w238
                shift-left: w235 -> [w248]
                n67 = call "E3631A_Voltage Controller.vi"("VISA resource name"=w250, "I_VDD(A)"=0.5, "Channel Controller"=w247, "Voltage 1"=0.0, "Voltage 2"=3.3, "error in (no error)"=w248, "I_3.3V (A)"=0.5) -> ("VISA resource name out"=w246:refnum<visa-resource-name>, "error out"=w241:errorcluster)  [unwired: 7 in]
                n68 = call "Delay T4.vi"("milliseconds to wait"=u32 100, "error in (no error)"=w241) -> ("error out"=w242:errorcluster)  [unwired: 9 in]
              }
              n69 = One Button Dialog(message="Calibration Completed....") -> ()  [unwired: 1 in, 1 out]
            }
          }
        }
      }
      n70 = call "Control Panel.vi"("error in (no error)"=w96, "Control Panel"="Control Panel") -> ("error out"=w93:errorcluster, "VPI"=w99:bool, "DVA"=w100:bool, "E-CAL"=w101:bool, "VSA"=w98:bool, "HD/CYC"=w102:bool, "HS"=w97:bool, "Verify Socket"=w103:bool)  [unwired: 2 in]
      "Verify Socket" <- w103
      "E-CAL" <- w101
      "VPI" <- w99
      "VSA" <- w98
      "HS" <- w97
      "HD/CYC" <- w102
      "DVA" <- w100
      n71 = Merge Errors(w93, w94) -> (w95:errorcluster)
      n72 = case shown="True" "Verify CP" {
        tunnel: [w147 w151] -> w105
        tunnel: w109 -> [w148 w154]
        tunnel: [w148 w152] -> w108
        tunnel: w95 -> [w147 w150]
        frame False {
        }
        frame True {
          w155 = T7 [enum."Voltage 2", enum."Voltage 3", enum."Voltage 1"] items=["Idle...", "Voltage 1", "Voltage 2", "Voltage 3"]
          # "Verify CP"
          n73 = for {
            tunnel: w154 -> [w168]
            tunnel: w155 -> [w166] mode=indexing
            shift-right: [w163] -> w153
            shift-left: w150 -> [w169]
            tunnel: [w161] -> w152
            n74 = local read "Set VDD"() -> (w165:dbl)
            n75 = call "E3631A_Voltage Controller.vi"("VISA resource name"=w168, "I_VDD(A)"=0.5, "Channel Controller"=w166, "Voltage 1"=w165, "Voltage 2"=3.3, "error in (no error)"=w169, "I_3.3V (A)"=0.5) -> ("VISA resource name out"=w161:refnum<visa-resource-name>, "error out"=w164:errorcluster)  [unwired: 7 in]
            n76 = call "Delay T4.vi"("milliseconds to wait"=u32 100, "error in (no error)"=w164) -> ("error out"=w163:errorcluster)  [unwired: 9 in]
          }
          n77 = Index Array(array=string[] ["074000", "074040", "07476F", "074776", "074800", "074820", "07413B", "074100", "07423B", "074200", "07433B", "074300"], index="CP Setting") -> (element=w156:string)
          n78 = call "WSVCAP SHL Host TL RFFE Write - Multiple DUTs - Common Data.vi"("Data Out"=w156, "error in"=w153, "Log (T)"=FALSE) -> ("error out"=w151:errorcluster)  [unwired: 12 in]
        }
      }
      n79 = Wait Until Next ms Multiple(millisecond multiple=u32 100) -> ()  [unwired: 1 out]
    }
    n80 = case shown="False" w73 {
      tunnel: w65 -> [w305 w1550]
      tunnel: [w290 w1550] -> w64
      tunnel: w67 -> [w304 w1548]
      tunnel: w66 -> [w296 w1549]
      tunnel: [w302 w1549] -> w78
      tunnel: [w300 w1548] -> w77
      tunnel: w75 -> [w293 w1547]
      tunnel: [w289 w1547] -> w74
      tunnel: "RFFE Slave Address" -> [w287 _]
      tunnel: [FALSE ("stop During HD/Cycles") FALSE ("stop During HD/Cycles")] -> _
      tunnel: w63 -> [w264 _]
      tunnel: w62 -> [w263 _]
      tunnel: w60 -> [w262 _]
      tunnel: w59 -> [w261 _]
      tunnel: w58 -> [w260 _]
      tunnel: w57 -> [w259 _]
      tunnel: w56 -> [w258 _]
      frame False {
        w267 = u32 100 ("milliseconds to wait")
        w301 = T7 [enum."Voltage 2", enum."Voltage 3", enum."Voltage 1"] items=["Idle...", "Voltage 1", "Voltage 2", "Voltage 3"]
        w303 = T7 [enum."Voltage 2", enum."Voltage 3", enum."Voltage 1"] items=["Idle...", "Voltage 1", "Voltage 2", "Voltage 3"]
        # "VSA"
        # "HS"
        # "HD/CYC"
        # "DVA"
        # "E-CAL"
        # "VPI"
        # "Verify Socket"
        n81 = for {
          tunnel: w305 -> [w1545]
          tunnel: w304 -> [w1544]
          tunnel: w303 -> [w1542] mode=indexing
          tunnel: [w1537] -> w298
          tunnel: [w1541] -> w288
          n82 = local read "Set VDD"() -> (w1540:dbl)
          n83 = call "E3631A_Voltage Controller.vi"("VISA resource name"=w1544, "I_VDD(A)"=0.5, "Channel Controller"=w1542, "Voltage 1"=w1540, "Voltage 2"=3.3, "error in (no error)"=w1545, "I_3.3V (A)"=0.5) -> ("VISA resource name out"=w1541:refnum<visa-resource-name>, "error out"=w1538:errorcluster)  [unwired: 7 in]
          n84 = call "Delay T4.vi"("milliseconds to wait"=u32 100, "error in (no error)"=w1538) -> ("error out"=w1537:errorcluster)  [unwired: 9 in]
        }
        n85 = call "WSVCAP SHL Host TL RFFE Write - Multiple DUTs - Common Data.vi"("Data Out"="074000", "error in"=w298, "Log (T)"=FALSE) -> ("error out"=w299:errorcluster)  [unwired: 12 in]
        n86 = local read "IDD Brd(uA)"() -> (w276:string)
        n87 = call "Delay T4.vi"("milliseconds to wait"=w267, "error in (no error)"=w299) -> ("error out"=w297:errorcluster)  [unwired: 9 in]
        n88 = case shown="False" "Serialize" {
          tunnel: [w307 w317] -> w266
          frame False {
            w306 = 36
            n89 = for {
              N: w306 -> [_]
              tunnel: [w312] -> w308 mode=indexing
              i -> [w316]
              n90 = Add(x="Start No", y=w316) -> (x+y=w314:i32)
              n91 = Number To Fractional String(number=w314, precision (6)=i16 0) -> (F-format string=w312:string)  [unwired: 2 in]
            }
            n92 = for {
              N: w306 -> [_]
              tunnel: w308 -> [w311]
              tunnel: [w310] -> w307 mode=indexing
              i -> [w309]
              n93 = Index Array(array=w311, index=w309) -> (element=w310:string)
            }
          }
          frame True {
            n94 = for {
              N: 36 -> [_]
              tunnel: "Serial Number" -> [w324]
              tunnel: [w322] -> w317 mode=indexing
              i -> [w321]
              n95 = Increment(x=w321) -> (x+1=w320:i32)
              n96 = Index Array(array=w324, index (row)=w320, index (col)=1 ("disabled index (col)")) -> (element=w322:string)
            }
          }
        }
        n97 = call "Ke2000 Single Reading.vi"("error in (no error)"=w297, "VISA resource name"=w296) -> ("error out"=w277:errorcluster, "VISA resource name out"=w295:refnum<visa-resource-name>, "uA"=w279:string)  [unwired: 5 in, 2 out]
        n98 = call "Substration.vi"("error in (no error)"=w277, "Input2"=w276, "Input1"=w279) -> ("error out"=w254:errorcluster, "In1 - In2"=w278:string)  [unwired: 7 in]
        "IDD Stdby(uA)" <- w278
        n99 = call "WSVCAP SHL Host TL RFFE Write - Multiple DUTs - Common Data.vi"("Data Out"="074040", "error in"=w254, "Log (T)"=FALSE) -> ("error out"=w253:errorcluster)  [unwired: 12 in]
        n100 = call "Delay T4.vi"("milliseconds to wait"=w267, "error in (no error)"=w253) -> ("error out"=w285:errorcluster)  [unwired: 9 in]
        n101 = case shown="True" w261 {
          tunnel: w285 -> [w342 w351]
          tunnel: [w341 w349] -> w283
          tunnel: ["DVA OFF" ("Data Out") "DVA ON" ("Data Out")] -> w284
          frame False {
            n102 = call "WSVCAP SHL Host TL RFFE Write - Multiple DUTs - Common Data.vi"("Data Out"="074820", "error in"=w342) -> ("error out"=w341:errorcluster)  [unwired: 13 in]
          }
          frame True {
            n103 = call "WSVCAP SHL Host TL RFFE Write - Multiple DUTs - Common Data.vi"("Data Out"="074800", "error in"=w351, "Log (T)"=FALSE) -> ("error out"=w347:errorcluster)  [unwired: 12 in]
            n104 = case shown="2" "CP with DVA ON" {
              selector: "CP with DVA ON" -> [w357 w362 w367 w372 w376]
              tunnel: string[] ["07442F", "074436", "074428", "074429", "07443B"] -> [w358 w363 w368 w373 w378]
              tunnel: [w356 w361 w366 w371 w377] -> w343
              tunnel: ["35.0" ("Data Out") "29.75" ("Data Out") "30.5" ("Data Out") "44.0" ("Data Out") "40.25" ("Data Out")] -> _
              tunnel: w347 -> [w354 w359 w364 w369 w374]
              tunnel: [w354 w359 w364 w369 w374] -> w346
              frame 0, Default {
                n105 = Index Array(array=w358, index=w357) -> (element=w356:string)
              }
              frame 2 {
                n106 = Index Array(array=w363, index=w362) -> (element=w361:string)
              }
              frame 3 {
                n107 = Index Array(array=w368, index=w367) -> (element=w366:string)
              }
              frame 4 {
                n108 = Index Array(array=w373, index=w372) -> (element=w371:string)
              }
              frame 1 {
                n109 = Index Array(array=w378, index=w376) -> (element=w377:string)
              }
            }
            n110 = call "WSVCAP SHL Host TL RFFE Write - Multiple DUTs - Common Data.vi"("Data Out"=w343, "error in"=w346, "Log (T)"=FALSE) -> ("error out"=w349:errorcluster)  [unwired: 12 in]
          }
        }
        n111 = Not(x=w258) -> (.not. x?=w265:bool)
        n112 = Number To Fractional String(number="Set VDD", precision (6)=i16 2) -> (F-format string=w281:string)  [unwired: 2 in]
        n113 = call "Delay T4.vi"("milliseconds to wait"=w267, "error in (no error)"=w283) -> ("error out"=w271:errorcluster)  [unwired: 9 in]
        n114 = case shown="True" w262 {
          tunnel: w271 -> [w328 w330]
          tunnel: [w325 w329] -> w270
          tunnel: ["CAL OFF" ("Data Out") "CAL ON" ("Data Out")] -> w272
          frame False {
            n115 = call "WSVCAP SHL Host TL RFFE Write - Multiple DUTs - Common Data.vi"("Data Out"="074044", "error in"=w328) -> ("error out"=w325:errorcluster)  [unwired: 13 in]
          }
          frame True {
            n116 = for {
              tunnel: string[] ["074900", "074920", "074900"] -> [w338] mode=indexing
              tunnel: w330 -> [w335]
              tunnel: [w334] -> w329
              n117 = call "WSVCAP SHL Host TL RFFE Write - Multiple DUTs - Common Data.vi"("Data Out"=w338, "error in"=w335, "Log (T)"=FALSE) -> ("error out"=w337:errorcluster)  [unwired: 12 in]
              n118 = call "Delay T4.vi"("milliseconds to wait"=u32 10, "error in (no error)"=w337) -> ("error out"=w334:errorcluster)  [unwired: 9 in]
            }
          }
        }
        n119 = for {
          N: 1 -> [_]
          tunnel: [w403] -> w302
          tunnel: w278 -> [w402]
          tunnel: w295 -> [w401]
          tunnel: "TMN DC\\CAP Data Log File Path" -> [w400]
          tunnel: w293 -> [w398]
          tunnel: [w397] -> w291
          tunnel: w288 -> [w379]
          tunnel: w263 -> [_]
          tunnel: w287 -> [w393]
          tunnel: w287 -> [w392]
          tunnel: w284 -> [w391]
          tunnel: w281 -> [w390]
          tunnel: [w389] -> w275
          tunnel: w272 -> [w388]
          tunnel: w270 -> [w387]
          tunnel: w261 -> [w386]
          tunnel: w264 -> [w384]
          tunnel: w260 -> [w383]
          tunnel: w265 -> [w382]
          tunnel: w259 -> [w381]
          tunnel: w266 -> [w380]
          tunnel: [w379] -> w255
          stop <- w385 stop-if-true
          n120 = while {
            tunnel: w400 -> [w616]
            tunnel: "Lot#" -> [w615]
            tunnel: "Wafer#" -> [w614]
            tunnel: w380 -> [w613]
            tunnel: "Test Program" -> [w612]
            tunnel: w380 -> [w611]
            tunnel: "Comment" -> [w610]
            tunnel: "Lot#" -> [w609]
            tunnel: "Wafer#" -> [w608]
            tunnel: w401 -> [w606]
            tunnel: [w607] -> w403
            tunnel: w402 -> [w605]
            tunnel: w398 -> [w603]
            tunnel: [w602] -> w397
            tunnel: [w523] -> w395
            tunnel: [w546] -> w394
            tunnel: w393 -> [w522]
            tunnel: w392 -> [w520]
            tunnel: w391 -> [w477]
            tunnel: w390 -> [w475]
            tunnel: [w455] -> w389
            tunnel: w388 -> [w461]
            tunnel: w387 -> [w460]
            tunnel: w386 -> [w459]
            tunnel: w384 -> [w452]
            tunnel: w383 -> [w451]
            tunnel: w382 -> [w446]
            tunnel: w381 -> [w440]
            i -> [w421]
            stop <- w552 stop-if-true
            n121 = case shown="False" "CP Sweep" {
              tunnel: [w620 w651] -> w474
              tunnel: [w619 w650] -> w409
              tunnel: [w618 w649] -> w473
              tunnel: w460 -> [w617 w652]
              tunnel: w421 -> [_ w648]
              frame False {
                n122 = case shown="4" "CP to HD/Cycle" {
                  selector: "CP to HD/Cycle" -> [w626 w631 w636 w641 w645]
                  tunnel: string[] ["07476F", "074776", "074765", "074769", "07477B"] -> [w627 w632 w637 w642 w647]
                  tunnel: [w625 w630 w635 w640 w646] -> w620
                  tunnel: ["35.0" ("Data Out") "27.5" ("Data Out") "30.5" ("Data Out") "44.0" ("Data Out") "40.25" ("Data Out")] -> w619
                  tunnel: [w623 w628 w633 w638 w643] -> w618
                  tunnel: w617 -> [w623 w628 w633 w638 w643]
                  frame 0, Default {
                    n123 = Index Array(array=w627, index=w626) -> (element=w625:string)
                  }
                  frame 2 {
                    n124 = Index Array(array=w632, index=w631) -> (element=w630:string)
                  }
                  frame 3 {
                    n125 = Index Array(array=w637, index=w636) -> (element=w635:string)
                  }
                  frame 4 {
                    n126 = Index Array(array=w642, index=w641) -> (element=w640:string)
                  }
                  frame 1 {
                    n127 = Index Array(array=w647, index=w645) -> (element=w646:string)
                  }
                }
              }
              frame True {
                n128 = case shown="1, Default" w648 {
                  tunnel: w652 -> [w655 w665]
                  tunnel: ["074040" w663] -> w651
                  tunnel: ["0" w662] -> w650
                  tunnel: w648 -> [_ w658]
                  tunnel: [w655 w660] -> w649
                  frame 0, 60 {
                  }
                  frame 1, Default {
                    n129 = call "WS1050 VPI CP Sweep Cmd.vi"("error in (no error)"=w665, "x"=23.0) -> ("error out"=w660:errorcluster, "Voltage Out"=w661:string[], "Cmd Out"=w664:string[])  [unwired: 5 in, 2 out]
                    n130 = Subtract(x=w658, y=1) -> (x-y=w656:i32)
                    n131 = Index Array(array=w664, index=w656) -> (element=w663:string)
                    n132 = Index Array(array=w661, index=w656) -> (element=w662:string)
                  }
                }
              }
            }
            n133 = flat-sequence {
              tunnel: [w710] -> w601
              tunnel: [w675] -> w600
              tunnel: w606 -> [w700]
              tunnel: w605 -> [w711]
              tunnel: [w711] -> w599
              tunnel: [w668] -> w598
              tunnel: [w668] -> w597
              tunnel: w473 -> [w709]
              tunnel: w421 -> [w666]
              tunnel: [w666] -> w551
              tunnel: ["Temperature"] -> w545
              tunnel: [w683] -> w540
              tunnel: [w682] -> w539
              tunnel: [w681] -> w538
              tunnel: [w686] -> w528
              tunnel: w522 -> [w708]
              tunnel: [w708] -> w521
              tunnel: w520 -> [_]
              tunnel: [w685] -> w508
              tunnel: [w684] -> w484
              tunnel: [w707] -> w478
              tunnel: w474 -> [w677]
              tunnel: ["NA" ("Data Out")] -> w465
              tunnel: w452 -> [w695]
              tunnel: w451 -> [w694]
              tunnel: [w694] -> w450
              tunnel: w446 -> [w693]
              tunnel: [w693] -> w445
              tunnel: w440 -> [w692]
              tunnel: [w692] -> w439
              tunnel: [w689] -> w434
              tunnel: ["Test Sequences"] -> w430
              tunnel: ["WS1050/51"] -> w425
              tunnel: w409 -> [w675]
              tunnel: [w675] -> w420
              tunnel: [w677] -> w416
              tunnel: [w762] -> w519
              tunnel: w601 -> [w765]
              tunnel: w600 -> [w770]
              tunnel: [w770] -> w518
              tunnel: w599 -> [w769]
              tunnel: w598 -> [w764]
              tunnel: w597 -> [w763]
              tunnel: [w754] -> w517
              tunnel: [w769] -> w516
              tunnel: [w764] -> w515
              tunnel: [w763] -> w514
              tunnel: w551 -> [w767]
              tunnel: [w767] -> w513
              tunnel: w545 -> [w766]
              tunnel: [w766] -> w512
              tunnel: [w765] -> w511
              tunnel: w540 -> [w761]
              tunnel: w539 -> [w747]
              tunnel: w538 -> [w748]
              tunnel: w528 -> [w760]
              tunnel: [w755] -> w510
              tunnel: w521 -> [w759]
              tunnel: [w745] -> w509
              tunnel: w508 -> [w745]
              tunnel: [w747] -> w507
              tunnel: w484 -> [w746]
              tunnel: [w746] -> w483
              tunnel: [w748] -> w481
              tunnel: w478 -> [w758]
              tunnel: [w757] -> w466
              tunnel: w465 -> [w757]
              tunnel: w450 -> [w753]
              tunnel: [w753] -> w449
              tunnel: w445 -> [w752]
              tunnel: [w752] -> w444
              tunnel: w439 -> [w751]
              tunnel: [w751] -> w438
              tunnel: w434 -> [w750]
              tunnel: [w749] -> w433
              tunnel: w430 -> [w744]
              tunnel: [w744] -> w429
              tunnel: w425 -> [w743]
              tunnel: [w743] -> w424
              tunnel: w420 -> [w742]
              tunnel: [w742] -> w419
              tunnel: w416 -> [w741]
              tunnel: [w741] -> w415
              tunnel: w519 -> [w893]
              tunnel: [w892] -> w506
              tunnel: w518 -> [w903]
              tunnel: [w903] -> w503
              tunnel: w517 -> [w884]
              tunnel: [w884] -> w501
              tunnel: w516 -> [w902]
              tunnel: [w902] -> w499
              tunnel: w515 -> [w901]
              tunnel: [w901] -> w497
              tunnel: w514 -> [w900]
              tunnel: [w900] -> w495
              tunnel: w513 -> [w899]
              tunnel: [w899] -> w493
              tunnel: w512 -> [w898]
              tunnel: [w898] -> w491
              tunnel: w511 -> [w897]
              tunnel: [w897] -> w489
              tunnel: [w889] -> w487
              tunnel: w510 -> [w888]
              tunnel: w509 -> [w895]
              tunnel: w507 -> [w894]
              tunnel: w483 -> [w881]
              tunnel: [w881] -> w482
              tunnel: w481 -> [w883]
              tunnel: [w883] -> w480
              tunnel: [w890] -> w479
              tunnel: [w891] -> w467
              tunnel: w466 -> [w891]
              tunnel: w449 -> [w887]
              tunnel: [w887] -> w448
              tunnel: w444 -> [w886]
              tunnel: [w886] -> w443
              tunnel: w438 -> [w885]
              tunnel: [w885] -> w437
              tunnel: w433 -> [w882]
              tunnel: w429 -> [w880]
              tunnel: [w882] -> w428
              tunnel: [w880] -> w427
              tunnel: w424 -> [w879]
              tunnel: [w879] -> w423
              tunnel: w419 -> [w878]
              tunnel: [w878] -> w418
              tunnel: w415 -> [w877]
              tunnel: [w877] -> w414
              tunnel: w506 -> [w1003]
              tunnel: [w1002] -> w505
              tunnel: [w998] -> w504
              tunnel: w503 -> [w1014]
              tunnel: [w1014] -> w502
              tunnel: w501 -> [w992]
              tunnel: [w992] -> w500
              tunnel: w499 -> [w1013]
              tunnel: [w1013] -> w498
              tunnel: w497 -> [w1012]
              tunnel: [w1012] -> w496
              tunnel: w495 -> [w1011]
              tunnel: [w1011] -> w494
              tunnel: w493 -> [w1010]
              tunnel: [w1010] -> w492
              tunnel: w491 -> [w1009]
              tunnel: [w1009] -> w490
              tunnel: w489 -> [w1008]
              tunnel: [w1008] -> w488
              tunnel: w487 -> [w1007]
              tunnel: [w1007] -> w486
              tunnel: [w990] -> w485
              tunnel: w482 -> [w1005]
              tunnel: w480 -> [w1004]
              tunnel: w479 -> [w997]
              tunnel: ["DeltaC Target Setting(pF)"] -> w476
              tunnel: [w1000] -> w468
              tunnel: w467 -> [w1000]
              tunnel: w459 -> [w999]
              tunnel: [w999] -> w458
              tunnel: w448 -> [w996]
              tunnel: [w996] -> w447
              tunnel: w443 -> [w995]
              tunnel: [w995] -> w442
              tunnel: w437 -> [w994]
              tunnel: [w994] -> w436
              tunnel: w428 -> [w993]
              tunnel: w427 -> [w991]
              tunnel: [w990] -> w426
              tunnel: w423 -> [w989]
              tunnel: [w989] -> w422
              tunnel: w418 -> [w988]
              tunnel: [w988] -> w417
              tunnel: w414 -> [w987]
              tunnel: [w987] -> w413
              tunnel: [w1147] -> w596
              tunnel: [w1118] -> w595
              tunnel: w505 -> [w1151]
              tunnel: w504 -> [w1129]
              tunnel: [w1138] -> w594
              tunnel: [w1129] -> w593
              tunnel: [w1150] -> w592
              tunnel: [w1149] -> w591
              tunnel: w502 -> [w1148]
              tunnel: [w1148] -> w590
              tunnel: w500 -> [w1138]
              tunnel: w498 -> [w1146]
              tunnel: [w1146] -> w589
              tunnel: w496 -> [w1142]
              tunnel: [w1142] -> w588
              tunnel: w494 -> [w1141]
              tunnel: [w1141] -> w587
              tunnel: w492 -> [w1139]
              tunnel: [w1139] -> w550
              tunnel: w490 -> [w1145]
              tunnel: [w1145] -> w544
              tunnel: w488 -> [w1144]
              tunnel: [w1143] -> w541
              tunnel: w486 -> [w1137]
              tunnel: [w1140] -> w537
              tunnel: [w1097] -> w536
              tunnel: [w1137] -> w531
              tunnel: w485 -> [w1136]
              tunnel: [w1123] -> w527
              tunnel: [w1122] -> w526
              tunnel: [w1121] -> w525
              tunnel: w476 -> [w1135]
              tunnel: [w1120] -> w469
              tunnel: w468 -> [w1120]
              tunnel: [w1119] -> w464
              tunnel: w458 -> [_]
              tunnel: w447 -> [w1116]
              tunnel: w442 -> [w1115]
              tunnel: [w1115] -> w441
              tunnel: w436 -> [w1114]
              tunnel: [w1114] -> w435
              tunnel: w426 -> [w1111]
              tunnel: w422 -> [w1110]
              tunnel: w417 -> [w1099]
              tunnel: w413 -> [w1100]
              tunnel: [w1099] -> w412
              tunnel: w596 -> [w1306]
              tunnel: [w1306] -> w586
              tunnel: [w1291] -> w585
              tunnel: [w1305] -> w584
              tunnel: w595 -> [w1304]
              tunnel: w594 -> [w1303]
              tunnel: w593 -> [w1302]
              tunnel: [w1303] -> w583
              tunnel: [w1302] -> w582
              tunnel: w592 -> [w1301]
              tunnel: [w1301] -> w581
              tunnel: w591 -> [w1300]
              tunnel: [w1300] -> w580
              tunnel: w590 -> [w1299]
              tunnel: [w1299] -> w579
              tunnel: w589 -> [w1298]
              tunnel: [w1298] -> w578
              tunnel: w588 -> [w1297]
              tunnel: [w1297] -> w577
              tunnel: w587 -> [w1296]
              tunnel: [w1296] -> w576
              tunnel: w603 -> [w1295]
              tunnel: [w1293] -> w575
              tunnel: [w1273] -> w574
              tunnel: [w1274] -> w573
              tunnel: [w1272] -> w572
              tunnel: w550 -> [w1289]
              tunnel: [w1289] -> w549
              tunnel: w544 -> [w1288]
              tunnel: [w1288] -> w543
              tunnel: w541 -> [w1305]
              tunnel: w537 -> [w1286]
              tunnel: w536 -> [w1287]
              tunnel: [w1287] -> w535
              tunnel: [w1286] -> w533
              tunnel: w531 -> [w1285]
              tunnel: [w1285] -> w530
              tunnel: w527 -> [_]
              tunnel: w526 -> [_]
              tunnel: w525 -> [_]
              tunnel: [w1270] -> w524
              tunnel: [w1268] -> w470
              tunnel: w469 -> [w1268]
              tunnel: w464 -> [w1271]
              tunnel: [w1271] -> w463
              tunnel: w441 -> [w1270]
              tunnel: w435 -> [w1267]
              tunnel: w412 -> [w1269]
              tunnel: [w1269] -> w411
              tunnel: w586 -> [w1387]
              tunnel: [w1387] -> w571
              tunnel: w585 -> [w1408]
              tunnel: [w1407] -> w570
              tunnel: w616 -> [w1409]
              tunnel: w615 -> [w1406]
              tunnel: w614 -> [w1405]
              tunnel: w613 -> [w1404]
              tunnel: [w1403] -> w569
              tunnel: w584 -> [w1397]
              tunnel: [w1397] -> w568
              tunnel: w583 -> [w1402]
              tunnel: w582 -> [w1401]
              tunnel: [w1402] -> w567
              tunnel: [w1401] -> w566
              tunnel: [w1395] -> w565
              tunnel: w581 -> [w1400]
              tunnel: [w1400] -> w564
              tunnel: w580 -> [w1399]
              tunnel: [w1399] -> w563
              tunnel: w579 -> [w1375]
              tunnel: [w1398] -> w562
              tunnel: [w1375] -> w561
              tunnel: w578 -> [w1396]
              tunnel: w577 -> [w1394]
              tunnel: w576 -> [w1393]
              tunnel: "File Name" -> [w1392]
              tunnel: w575 -> [w1391]
              tunnel: [w1391] -> w560
              tunnel: w574 -> [w1390]
              tunnel: [w1390] -> w559
              tunnel: [w1389] -> w558
              tunnel: w573 -> [w1389]
              tunnel: w572 -> [w1388]
              tunnel: [w1388] -> w557
              tunnel: w549 -> [w1374]
              tunnel: [w1374] -> w547
              tunnel: w543 -> [w1386]
              tunnel: [w1386] -> w542
              tunnel: w535 -> [w1385]
              tunnel: [w1385] -> w534
              tunnel: w533 -> [w1384]
              tunnel: [w1384] -> w532
              tunnel: w530 -> [w1383]
              tunnel: [w1383] -> w529
              tunnel: w524 -> [w1382]
              tunnel: "NA" ("Data Out") -> [w1381]
              tunnel: [w1381] -> w472
              tunnel: [w1380] -> w471
              tunnel: w470 -> [w1380]
              tunnel: w463 -> [w1379]
              tunnel: [w1379] -> w462
              tunnel: ["Freq(Hz)"] -> w432
              tunnel: ["Board#"] -> w431
              tunnel: w411 -> [w1376]
              tunnel: [w1376] -> w410
              tunnel: w571 -> [w1476]
              tunnel: w570 -> [w1475]
              tunnel: w616 -> [w1444]
              tunnel: w612 -> [w1470]
              tunnel: w611 -> [w1473]
              tunnel: w610 -> [w1469]
              tunnel: w609 -> [w1472]
              tunnel: w608 -> [w1468]
              tunnel: w569 -> [w1471]
              tunnel: [w1476] -> w554
              tunnel: [w1474] -> w555
              tunnel: w568 -> [w1466]
              tunnel: [w1466] -> w556
              tunnel: w567 -> [w1465]
              tunnel: w566 -> [w1452]
              tunnel: w565 -> [w1464]
              tunnel: w564 -> [w1463]
              tunnel: w563 -> [w1454]
              tunnel: w562 -> [w1462]
              tunnel: w561 -> [w1461]
              tunnel: "File Name" -> [w1437]
              tunnel: w560 -> [w1460]
              tunnel: [w1460] -> w553
              tunnel: w559 -> [w1459]
              tunnel: w558 -> [w1458]
              tunnel: w557 -> [w1457]
              tunnel: [w1440] -> w548
              tunnel: w547 -> [w1440]
              tunnel: w542 -> [w1456]
              tunnel: w534 -> [w1455]
              tunnel: w532 -> [w1453]
              tunnel: w529 -> [w1451]
              tunnel: w477 -> [w1450]
              tunnel: w461 -> [w1449]
              tunnel: w475 -> [w1448]
              tunnel: w472 -> [w1447]
              tunnel: w471 -> [w1446]
              tunnel: w462 -> [w1445]
              tunnel: [w1442] -> w457
              tunnel: [w1433] -> w453
              tunnel: w432 -> [w1432]
              tunnel: w431 -> [w1430]
              tunnel: w410 -> [w1429]
              tunnel: [w1495] -> w607
              tunnel: [w1496] -> w523
              tunnel: w556 -> [w1495]
              tunnel: w555 -> [w1488]
              tunnel: w554 -> [w1496]
              tunnel: w553 -> [w1490]
              tunnel: [w1490] -> w602
              tunnel: w548 -> [w1484]
              tunnel: [w1483] -> w546
              tunnel: [w1481] -> w454
              tunnel: w457 -> [w1487]
              tunnel: w453 -> [w1485]
              frame #0 {
                n134 = call "WSVCAP SHL Host TL RFFE Write - Multiple DUTs - Common Data.vi"("Data Out"=w677, "error in"=w709, "Log (T)"=FALSE) -> ("error out"=w696:errorcluster)  [unwired: 12 in]
                n135 = for {
                  tunnel: string[] ["0760", "0767", "0768"] -> [w733] mode=indexing
                  tunnel: [w729] -> w698 mode=indexing
                  tunnel: w696 -> [w727]
                  tunnel: [w726] -> w697
                  i -> [w732]
                  n136 = call "Delay T4.vi"("milliseconds to wait"=u32 10, "error in (no error)"=w727) -> ("error out"=w734:errorcluster)  [unwired: 9 in]
                  n137 = call "WSVCAP SHL Host TL RFFE Read - Multiple DUTs - Common Data.vi"("Data Out"=w733, "error in"=w734, "Log (T)"=FALSE) -> ("RFFE Data In"=w731:string[], "error out"=w726:errorcluster)  [unwired: 11 in]
                  n138 = Index Array(array=w731, index=w732) -> (element=w728:string)
                  n139 = String Subset(string=w728, offset (0)=0) -> (substring=w729:string)  [unwired: 1 in]
                }
                "RB Reg for HD/Cycle" <- w698
                n140 = Not(x=w695) -> ()  [unwired: 1 out]
                n141 = local read "IDD Brd(uA)"() -> (w706:string)
                n142 = call "Delay T4.vi"("milliseconds to wait"=u32 100, "error in (no error)"=w697) -> ("error out"=w702:errorcluster)  [unwired: 9 in]
                n143 = call "Ke2000 Single Reading.vi"("error in (no error)"=w702, "VISA resource name"=w700) -> ("error out"=w704:errorcluster, "VISA resource name out"=w680:refnum<visa-resource-name>, "uA"=w705:string)  [unwired: 5 in, 2 out]
                n144 = call "Substration.vi"("error in (no error)"=w704, "Input2"=w706, "Input1"=w705) -> ("error out"=w674:errorcluster, "In1 - In2"=→"IDD_HD/CYC (uA)":string)  [unwired: 7 in]
                n145 = case shown="0, 60" w666 {
                  tunnel: w674 -> [w716 w718 w721]
                  tunnel: [w712 w718 w724] -> w667
                  frame 0, 60 {
                    n146 = call "Delay T4.vi"("milliseconds to wait"=u32 10, "error in (no error)"=w716) -> ("error out"=w715:errorcluster)  [unwired: 9 in]
                    n147 = call "WSVCAP SHL Host TL RFFE Write - Multiple DUTs - Common Data.vi"("Data Out"="070201000000", "error in"=w715, "Log (T)"=FALSE) -> ("error out"=w712:errorcluster)  [unwired: 12 in]
                  }
                  frame 2, Default {
                  }
                  frame 1 {
                    n148 = call "Delay T4.vi"("milliseconds to wait"=u32 10, "error in (no error)"=w721) -> ("error out"=w720:errorcluster)  [unwired: 9 in]
                    n149 = call "WSVCAP SHL Host TL RFFE Write - Multiple DUTs - Common Data.vi"("Data Out"="0702013B3B3B", "error in"=w720, "Log (T)"=FALSE) -> ("error out"=w724:errorcluster)  [unwired: 12 in]
                  }
                }
                n150 = flat-sequence {
                  tunnel: w691 -> [w736]
                  tunnel: [w736] -> w688
                  frame #0 {
                    w737 = "0" ("NOM IDD OFF(uA)")
                    w738 = string[] []
                    w739 = string[][] []
                    n151 = local write "NOM IDD ON (uA)"(w737) -> ()
                    n152 = local write "Total Delta C1(pF)"(w738) -> ()
                    n153 = local write "Total Delta C2(pF)"(w738) -> ()
                    n154 = local write "Total Delta C3(pF)"(w738) -> ()
                    n155 = local write "Current EFuse Read back"(w738) -> ()
                    n156 = local write "RB Reg for HD/Cycle"(w738) -> ()
                    n157 = local write "NOM IDD OFF(uA)"(w737) -> ()
                    n158 = local write "VSA_V3"(w739) -> ()
                    n159 = local write "VSA_V1"(w739) -> ()
                    n160 = local write "VSA_V2"(w739) -> ()
                    n161 = local write "VPI C1"(w739) -> ()
                    n162 = local write "VPI C2"(w739) -> ()
                    n163 = local write "VPI C3"(w739) -> ()
                    n164 = local write "% Delta C"(w739) -> ()
                    n165 = local write "40V_3"(w739) -> ()
                    n166 = local write "40V_2"(w739) -> ()
                    n167 = local write "40V_1"(w739) -> ()
                  }
                }
                n168 = local read "IDD Brd(uA)"() -> (w669:string)
                n169 = call "Delay T4.vi"("milliseconds to wait"=u32 100, "error in (no error)"=w667) -> ("error out"=w672:errorcluster)  [unwired: 9 in]
                n170 = call "Ke2000 Single Reading.vi"("error in (no error)"=w672, "VISA resource name"=w680) -> ("error out"=w671:errorcluster, "VISA resource name out"=w710:refnum<visa-resource-name>, "uA"=w670:string)  [unwired: 5 in, 2 out]
                n171 = call "Substration.vi"("error in (no error)"=w671, "Input2"=w669, "Input1"=w670) -> ("error out"=w691:errorcluster, "In1 - In2"=w668:string)  [unwired: 7 in]
                n172 = local read "Clock Rate (Hz)"() -> (w707:dbl)
                n173 = call "Multi Dut Cmd_Header Setting.vi"("error in (no error)"=w688, "Test Seq"="Test Sequences", "WS1050/51"="WS1050/51") -> ("error out"=w689:errorcluster, "Cmd 3"=w681:string[], "Name 3"=w684:string[], "Cmd 2"=w682:string[], "Name 2"=w685:string[], "Cmd 1"=w683:string[], "Name 1"=w686:string[])  [unwired: 1 in, 1 out]
              }
              frame #1 {
                w749 = FALSE ("Log (T)")
                n174 = call "WSVCAP SHL Host TL RFFE Configure.vi"("RFFE Slave Address"=w759, "Clock Rate (Hz)"=w758, "error in"=w750) -> ("Actual Rate (Hz)"=w768:dbl, "error out"=w756:errorcluster)  [unwired: 11 in]
                n175 = local write "AR  Measurent(Hz)"(w768) -> ()
                n176 = Array Size(array=w760) -> (size(s)=w771:i32)
                n177 = case shown="True" FALSE {
                  tunnel: w771 -> [_ w784]
                  tunnel: [_ w783] -> w762
                  tunnel: w761 -> [_ w782]
                  tunnel: w760 -> [_ w781]
                  tunnel: w756 -> [w773 w780]
                  tunnel: [w773 w779] -> w755
                  tunnel: [string[][] [] w778] -> w754
                  tunnel: w749 -> [_ w777]
                  tunnel: w744 -> [_ w775]
                  tunnel: w742 -> [_ w774]
                  frame False {
                  }
                  frame True {
                    n178 = case shown="0, Default" w775 {
                      tunnel: w784 -> [w793 w825 w854]
                      tunnel: [w792 w824 w853] -> w783
                      tunnel: w782 -> [w791 w823 w852]
                      tunnel: w781 -> [w790 w822 w851]
                      tunnel: w780 -> [w789 w821 w850]
                      tunnel: [w788 w820 w849] -> w779
                      tunnel: w777 -> [w787 w819 w848]
                      tunnel: [w786 w818 w847] -> w776
                      tunnel: w774 -> [w785 _ _]
                      frame 0, Default {
                        n179 = for {
                          N: w793 -> [_]
                          tunnel: w791 -> [w813]
                          tunnel: [w794] -> w792
                          tunnel: [w810] -> w786 mode=indexing
                          tunnel: w790 -> [w811]
                          tunnel: w789 -> [w800]
                          tunnel: [w802] -> w788
                          tunnel: w787 -> [w801]
                          tunnel: w785 -> [w795]
                          i -> [w809]
                          stop <- w794 stop-if-true
                          n180 = Index Array(array=w813, index=w809) -> (element=w812:string)
                          n181 = Index Array(array=w811, index=w809) -> (element=w797:string)
                          n182 = call <vilib>:"Space Constant.vi"() -> ("String"=w796:string)
                          n183 = call "WSVCAP SHL Host TL RFFE Write - Multiple DUTs - Common Data.vi"("Data Out"=w812, "error in"=w800, "Log (T)"=FALSE) -> ("error out"=w804:errorcluster)  [unwired: 12 in]
                          n184 = Concatenate Strings(w797, w796, w795) -> (w798:string)
                          n185 = call "Delay T4.vi"("milliseconds to wait"=u32 10, "error in (no error)"=w804) -> ("error out"=w808:errorcluster)  [unwired: 9 in]
                          n186 = call "WS1050 AD7747 READ 36 DUT.vi"("error in"=w808, "Log (T)"=w801, "DUT Mask Mode (All)"=WSVCAP_SHL_I2C_DUT_Mask_Mode_Enum."C1") -> ("error out"=w806:errorcluster, "AD7747 Values"=w807:string[][])  [unwired: 7 in]
                          n187 = local write "STATUS"(w798) -> ()
                          n188 = for {
                            tunnel: w807 -> [w816] mode=indexing
                            tunnel: w806 -> [w817]
                            tunnel: [w817] -> w802
                            tunnel: [w814] -> w810 mode=indexing
                            n189 = Index Array(array=w816, index=1) -> (element=w814:string)
                          }
                          n190 = Unbundle By Name(w802) -> ("status"=w794:bool)
                        }
                      }
                      frame 1 {
                        n191 = for {
                          N: w825 -> [_]
                          tunnel: w823 -> [w842]
                          tunnel: [w826] -> w824
                          tunnel: [w838] -> w818 mode=indexing
                          tunnel: w822 -> [w840]
                          tunnel: w821 -> [w828]
                          tunnel: [w830] -> w820
                          tunnel: w819 -> [w829]
                          i -> [w837]
                          stop <- w826 stop-if-true
                          n192 = Index Array(array=w842, index=w837) -> (element=w841:string)
                          n193 = Index Array(array=w840, index=w837) -> (element=w839:string)
                          n194 = local write "STATUS"(w839) -> ()
                          n195 = call "WSVCAP SHL Host TL RFFE Write - Multiple DUTs - Common Data.vi"("Data Out"=w841, "error in"=w828, "Log (T)"=FALSE) -> ("error out"=w832:errorcluster)  [unwired: 12 in]
                          n196 = call "Delay T4.vi"("milliseconds to wait"=u32 10, "error in (no error)"=w832) -> ("error out"=w836:errorcluster)  [unwired: 9 in]
                          n197 = call "WS1050 AD7747 READ 36 DUT.vi"("error in"=w836, "Log (T)"=w829, "DUT Mask Mode (All)"=WSVCAP_SHL_I2C_DUT_Mask_Mode_Enum."C2") -> ("error out"=w834:errorcluster, "AD7747 Values"=w835:string[][])  [unwired: 7 in]
                          n198 = for {
                            tunnel: w835 -> [w845] mode=indexing
                            tunnel: w834 -> [w846]
                            tunnel: [w846] -> w830
                            tunnel: [w843] -> w838 mode=indexing
                            n199 = Index Array(array=w845, index=3) -> (element=w843:string)
                          }
                          n200 = Unbundle By Name(w830) -> ("status"=w826:bool)
                        }
                      }
                      frame 2 {
                        n201 = for {
                          N: w854 -> [_]
                          tunnel: w852 -> [w871]
                          tunnel: [w855] -> w853
                          tunnel: [w867] -> w847 mode=indexing
                          tunnel: w851 -> [w869]
                          tunnel: w850 -> [w857]
                          tunnel: [w859] -> w849
                          tunnel: w848 -> [w858]
                          i -> [w866]
                          stop <- w855 stop-if-true
                          n202 = Index Array(array=w871, index=w866) -> (element=w870:string)
                          n203 = Index Array(array=w869, index=w866) -> (element=w868:string)
                          n204 = local write "STATUS"(w868) -> ()
                          n205 = call "WSVCAP SHL Host TL RFFE Write - Multiple DUTs - Common Data.vi"("Data Out"=w870, "error in"=w857, "Log (T)"=FALSE) -> ("error out"=w861:errorcluster)  [unwired: 12 in]
                          n206 = call "Delay T4.vi"("milliseconds to wait"=u32 10, "error in (no error)"=w861) -> ("error out"=w865:errorcluster)  [unwired: 9 in]
                          n207 = call "WS1050 AD7747 READ 36 DUT.vi"("error in"=w865, "Log (T)"=w858, "DUT Mask Mode (All)"=WSVCAP_SHL_I2C_DUT_Mask_Mode_Enum."C3") -> ("error out"=w863:errorcluster, "AD7747 Values"=w864:string[][])  [unwired: 7 in]
                          n208 = for {
                            tunnel: w864 -> [w874] mode=indexing
                            tunnel: w863 -> [w875]
                            tunnel: [w875] -> w859
                            tunnel: [w872] -> w867 mode=indexing
                            n209 = Index Array(array=w874, index=5) -> (element=w872:string)
                          }
                          n210 = Unbundle By Name(w859) -> ("status"=w855:bool)
                        }
                      }
                    }
                    n211 = Transpose 2D Array(2D array=w776) -> (transposed array=w778:string[][])
                    "40V_1" <- w778
                  }
                }
                "NOM IDD ON (uA)" <- w764
                "NOM IDD OFF(uA)" <- w763
              }
              frame #2 {
                n212 = Array Size(array=w895) -> (size(s)=w896:i32)
                n213 = case shown="False" FALSE {
                  tunnel: w896 -> [_ w917]
                  tunnel: w895 -> [_ w916]
                  tunnel: w894 -> [_ w915]
                  tunnel: w893 -> [_ w914]
                  tunnel: [_ w913] -> w892
                  tunnel: [w905 w912] -> w890
                  tunnel: [string[][] [] w911] -> w889
                  tunnel: w888 -> [w905 w910]
                  tunnel: w882 -> [_ w909]
                  tunnel: w880 -> [_ w907]
                  tunnel: w878 -> [_ w906]
                  frame False {
                  }
                  frame True {
                    n214 = case shown="0, 2, Default" w907 {
                      tunnel: w917 -> [w927 w962]
                      tunnel: w916 -> [w926 w961]
                      tunnel: w915 -> [w925 w960]
                      tunnel: w914 -> [w924 w959]
                      tunnel: [w923 w958] -> w913
                      tunnel: [w922 w957] -> w912
                      tunnel: w910 -> [w921 w956]
                      tunnel: w909 -> [w920 w955]
                      tunnel: [w919 w954] -> w908
                      tunnel: w906 -> [w918 _]
                      frame 0, 2, Default {
                        n215 = for {
                          N: w927 -> [_]
                          tunnel: w925 -> [w949]
                          tunnel: w924 -> [w947]
                          tunnel: [w946] -> w923
                          tunnel: [w943] -> w919 mode=indexing
                          tunnel: w926 -> [w944]
                          tunnel: w921 -> [w933]
                          tunnel: [w935] -> w922
                          tunnel: w920 -> [w934]
                          tunnel: w918 -> [w928]
                          i -> [w942]
                          stop <- w946 stop-if-true
                          n216 = Index Array(array=w949, index=w942) -> (element=w945:string)
                          n217 = Index Array(array=w944, index=w942) -> (element=w929:string)
                          n218 = call <vilib>:"Space Constant.vi"() -> ("String"=w930:string)
                          n219 = call "WSVCAP SHL Host TL RFFE Write - Multiple DUTs - Common Data.vi"("Data Out"=w945, "error in"=w933, "Log (T)"=FALSE) -> ("error out"=w937:errorcluster)  [unwired: 12 in]
                          n220 = Concatenate Strings(w929, w930, w928) -> (w931:string)
                          n221 = call "Delay T4.vi"("milliseconds to wait"=u32 10, "error in (no error)"=w937) -> ("error out"=w941:errorcluster)  [unwired: 9 in]
                          n222 = call "WS1050 AD7747 READ 36 DUT.vi"("error in"=w941, "Log (T)"=w934, "DUT Mask Mode (All)"=WSVCAP_SHL_I2C_DUT_Mask_Mode_Enum."C2") -> ("error out"=w939:errorcluster, "AD7747 Values"=w940:string[][])  [unwired: 7 in]
                          n223 = local write "STATUS"(w931) -> ()
                          n224 = for {
                            tunnel: w940 -> [w952] mode=indexing
                            tunnel: w939 -> [w953]
                            tunnel: [w953] -> w935
                            tunnel: [w950] -> w943 mode=indexing
                            n225 = Index Array(array=w952, index=3) -> (element=w950:string)
                          }
                          n226 = Unbundle By Name(w935) -> ("status"=w948:bool)
                          n227 = Or(x=w948, y=w947) -> (x .or. y?=w946:bool)
                        }
                      }
                      frame 1 {
                        n228 = for {
                          N: w962 -> [_]
                          tunnel: w960 -> [w981]
                          tunnel: w959 -> [w979]
                          tunnel: [w978] -> w958
                          tunnel: [w974] -> w954 mode=indexing
                          tunnel: w961 -> [w976]
                          tunnel: w956 -> [w964]
                          tunnel: [w966] -> w957
                          tunnel: w955 -> [w965]
                          i -> [w973]
                          stop <- w978 stop-if-true
                          n229 = Index Array(array=w981, index=w973) -> (element=w977:string)
                          n230 = Index Array(array=w976, index=w973) -> (element=w975:string)
                          n231 = call "WSVCAP SHL Host TL RFFE Write - Multiple DUTs - Common Data.vi"("Data Out"=w977, "error in"=w964, "Log (T)"=FALSE) -> ("error out"=w968:errorcluster)  [unwired: 12 in]
                          n232 = local write "STATUS"(w975) -> ()
                          n233 = call "Delay T4.vi"("milliseconds to wait"=u32 10, "error in (no error)"=w968) -> ("error out"=w972:errorcluster)  [unwired: 9 in]
                          n234 = call "WS1050 AD7747 READ 36 DUT.vi"("error in"=w972, "Log (T)"=w965, "DUT Mask Mode (All)"=WSVCAP_SHL_I2C_DUT_Mask_Mode_Enum."C1") -> ("error out"=w970:errorcluster, "AD7747 Values"=w971:string[][])  [unwired: 7 in]
                          n235 = for {
                            tunnel: w971 -> [w984] mode=indexing
                            tunnel: w970 -> [w985]
                            tunnel: [w985] -> w966
                            tunnel: [w982] -> w974 mode=indexing
                            n236 = Index Array(array=w984, index=1) -> (element=w982:string)
                          }
                          n237 = Unbundle By Name(w966) -> ("status"=w980:bool)
                          n238 = Or(x=w980, y=w979) -> (x .or. y?=w978:bool)
                        }
                      }
                    }
                    n239 = Transpose 2D Array(2D array=w908) -> (transposed array=w911:string[][])
                    "40V_2" <- w911
                  }
                }
              }
              frame #3 {
                n240 = Array Size(array=w1005) -> (size(s)=w1006:i32)
                n241 = case shown="False" FALSE {
                  tunnel: w1006 -> [_ w1028]
                  tunnel: w1005 -> [_ w1027]
                  tunnel: w1004 -> [_ w1026]
                  tunnel: w1003 -> [_ w1025]
                  tunnel: [_ w1024] -> w1002
                  tunnel: [string[][] [] w1023] -> w998
                  tunnel: w997 -> [w1016 w1022]
                  tunnel: w993 -> [_ w1021]
                  tunnel: w991 -> [_ w1019]
                  tunnel: [w1016 w1018] -> w990
                  tunnel: w988 -> [_ w1017]
                  frame False {
                  }
                  frame True {
                    n242 = case shown="0, 1, Default" w1019 {
                      tunnel: w1028 -> [w1038 w1073]
                      tunnel: w1027 -> [w1037 w1072]
                      tunnel: w1026 -> [w1036 w1071]
                      tunnel: w1025 -> [w1035 w1070]
                      tunnel: [w1034 w1069] -> w1024
                      tunnel: w1022 -> [w1033 w1068]
                      tunnel: [w1032 w1067] -> w1018
                      tunnel: w1021 -> [w1031 w1066]
                      tunnel: [w1030 w1065] -> w1020
                      tunnel: w1017 -> [w1029 _]
                      frame 0, 1, Default {
                        n243 = for {
                          N: w1038 -> [_]
                          tunnel: w1036 -> [w1060]
                          tunnel: w1035 -> [w1058]
                          tunnel: [w1057] -> w1034
                          tunnel: [w1054] -> w1030 mode=indexing
                          tunnel: w1037 -> [w1055]
                          tunnel: w1033 -> [w1044]
                          tunnel: [w1046] -> w1032
                          tunnel: w1031 -> [w1045]
                          tunnel: w1029 -> [w1039]
                          i -> [w1053]
                          stop <- w1057 stop-if-true
                          n244 = Index Array(array=w1060, index=w1053) -> (element=w1056:string)
                          n245 = Index Array(array=w1055, index=w1053) -> (element=w1041:string)
                          n246 = call <vilib>:"Space Constant.vi"() -> ("String"=w1040:string)
                          n247 = call "WSVCAP SHL Host TL RFFE Write - Multiple DUTs - Common Data.vi"("Data Out"=w1056, "error in"=w1044, "Log (T)"=FALSE) -> ("error out"=w1048:errorcluster)  [unwired: 12 in]
                          n248 = call "Delay T4.vi"("milliseconds to wait"=u32 10, "error in (no error)"=w1048) -> ("error out"=w1052:errorcluster)  [unwired: 9 in]
                          n249 = Concatenate Strings(w1041, w1040, w1039) -> (w1042:string)
                          n250 = call "WS1050 AD7747 READ 36 DUT.vi"("error in"=w1052, "Log (T)"=w1045, "DUT Mask Mode (All)"=WSVCAP_SHL_I2C_DUT_Mask_Mode_Enum."C3") -> ("error out"=w1050:errorcluster, "AD7747 Values"=w1051:string[][])  [unwired: 7 in]
                          n251 = for {
                            tunnel: w1051 -> [w1063] mode=indexing
                            tunnel: w1050 -> [w1064]
                            tunnel: [w1064] -> w1046
                            tunnel: [w1061] -> w1054 mode=indexing
                            n252 = Index Array(array=w1063, index=5) -> (element=w1061:string)
                          }
                          n253 = Unbundle By Name(w1046) -> ("status"=w1059:bool)
                          n254 = local write "STATUS"(w1042) -> ()
                          n255 = Or(x=w1059, y=w1058) -> (x .or. y?=w1057:bool)
                        }
                      }
                      frame 2 {
                        n256 = for {
                          N: w1073 -> [_]
                          tunnel: w1071 -> [w1092]
                          tunnel: w1070 -> [w1090]
                          tunnel: [w1089] -> w1069
                          tunnel: [w1085] -> w1065 mode=indexing
                          tunnel: w1072 -> [w1087]
                          tunnel: w1068 -> [w1075]
                          tunnel: [w1077] -> w1067
                          tunnel: w1066 -> [w1076]
                          i -> [w1084]
                          stop <- w1089 stop-if-true
                          n257 = Index Array(array=w1092, index=w1084) -> (element=w1088:string)
                          n258 = Index Array(array=w1087, index=w1084) -> (element=w1086:string)
                          n259 = local write "STATUS"(w1086) -> ()
                          n260 = call "WSVCAP SHL Host TL RFFE Write - Multiple DUTs - Common Data.vi"("Data Out"=w1088, "error in"=w1075, "Log (T)"=FALSE) -> ("error out"=w1079:errorcluster)  [unwired: 12 in]
                          n261 = call "Delay T4.vi"("milliseconds to wait"=u32 10, "error in (no error)"=w1079) -> ("error out"=w1083:errorcluster)  [unwired: 9 in]
                          n262 = call "WS1050 AD7747 READ 36 DUT.vi"("error in"=w1083, "Log (T)"=w1076, "DUT Mask Mode (All)"=WSVCAP_SHL_I2C_DUT_Mask_Mode_Enum."C1") -> ("error out"=w1081:errorcluster, "AD7747 Values"=w1082:string[][])  [unwired: 7 in]
                          n263 = for {
                            tunnel: w1082 -> [w1095] mode=indexing
                            tunnel: w1081 -> [w1096]
                            tunnel: [w1096] -> w1077
                            tunnel: [w1093] -> w1085 mode=indexing
                            n264 = Index Array(array=w1095, index=1) -> (element=w1093:string)
                          }
                          n265 = Unbundle By Name(w1077) -> ("status"=w1091:bool)
                          n266 = Or(x=w1091, y=w1090) -> (x .or. y?=w1089:bool)
                        }
                      }
                    }
                    n267 = Transpose 2D Array(2D array=w1020) -> (transposed array=w1023:string[][])
                    "40V_3" <- w1023
                  }
                }
              }
              frame #4 {
                # "VPI Testing @ 35V"
                n268 = call "WS1050 Delta C Calculation.vi"("error in (no error)"=w1136, "DCap Target(pF)"=w1135, "Input"=w1138) -> ("error out"=w1133:errorcluster, "Total Bank Delta C(pF)"=w1126:string[], "% Bank DeltaC"=w1130:string[])  [unwired: 3 in, 3 out]
                n269 = call "WS1050 Delta C Calculation.vi"("error in (no error)"=w1136, "DCap Target(pF)"=w1135, "Input"=w1137) -> ("error out"=w1134:errorcluster, "Total Bank Delta C(pF)"=w1125:string[], "% Bank DeltaC"=w1128:string[])  [unwired: 3 in, 3 out]
                n270 = call "WS1050 Delta C Calculation.vi"("error in (no error)"=w1136, "DCap Target(pF)"=w1135, "Input"=w1129) -> ("error out"=w1132:errorcluster, "Total Bank Delta C(pF)"=w1124:string[], "% Bank DeltaC"=w1127:string[])  [unwired: 3 in, 3 out]
                n271 = call "WS1050_51 VPI Header CV Curve.vi"("error in (no error)"=w1111, "WS1050/51"=w1110, "VPI_Cmd"="VPI_Cmd", "VPI Name"="VPI Name") -> ("error out"=w1103:errorcluster, "Cmd_3"=w1104:string[], "VPI_3"=w1107:string[], "VPI Header"=w1097:string[], "Cmd_2"=w1105:string[], "VPI_2"=w1108:string[], "Cmd_1"=w1106:string[], "VPI_1"=w1109:string[])
                n272 = Merge Errors(w1133, w1134, w1132) -> (w1131:errorcluster)
                n273 = case shown="1, Default" w1139 {
                  tunnel: w1131 -> [w1159 w1167]
                  tunnel: [w1159 w1167] -> w1102
                  tunnel: w1130 -> [w1155 w1163]
                  tunnel: w1128 -> [w1154 w1162]
                  tunnel: w1127 -> [w1153 w1161]
                  tunnel: w1126 -> [w1158 w1166]
                  tunnel: [w1158 w1166] -> w1123
                  tunnel: w1125 -> [w1157 w1165]
                  tunnel: [w1157 w1165] -> w1122
                  tunnel: w1124 -> [w1156 w1164]
                  tunnel: [w1156 w1164] -> w1121
                  frame 0 {
                    n274 = Build Array(w1155, w1154, w1153) -> (→"% Delta C_T0":string[][])
                  }
                  frame 1, Default {
                    n275 = Build Array(w1163, w1162, w1161) -> (→"% Delta C":string[][])
                  }
                }
                "Total Delta C1(pF)" <- w1123
                "Total Delta C2(pF)" <- w1122
                "Total Delta C3(pF)" <- w1121
                n276 = Merge Errors(w1103, w1102) -> (w1101:errorcluster)
                n277 = case shown="True" w1116 {
                  tunnel: w1151 -> [w1170 w1196]
                  tunnel: [w1169 w1188] -> w1098
                  tunnel: [w1168 w1177] -> w1150
                  tunnel: [w1168 w1175] -> w1149
                  tunnel: [w1170 w1189] -> w1147
                  tunnel: w1144 -> [w1172 w1197]
                  tunnel: [w1172 w1197] -> w1143
                  tunnel: w1106 -> [_ w1195]
                  tunnel: w1105 -> [_ w1192]
                  tunnel: w1104 -> [_ w1190]
                  tunnel: [w1168 w1176] -> w1140
                  tunnel: w1109 -> [_ w1194]
                  tunnel: w1108 -> [_ w1193]
                  tunnel: w1107 -> [_ w1191]
                  tunnel: ["NA" ("string") w1174] -> w1119
                  tunnel: w1101 -> [w1169 w1173]
                  tunnel: w1099 -> [_ w1174]
                  tunnel: w1100 -> [_ _]
                  frame False {
                    w1168 = string[][] []
                  }
                  frame True {
                    n278 = Array Size(array=w1194) -> (size(s)=w1178:i32)
                    n279 = for {
                      N: w1178 -> [_]
                      tunnel: w1195 -> [w1262]
                      tunnel: w1196 -> [w1260]
                      tunnel: [w1259] -> w1185
                      tunnel: [w1258] -> w1187 mode=indexing
                      tunnel: w1194 -> [w1257]
                      tunnel: w1173 -> [w1244]
                      tunnel: [w1250] -> w1180
                      tunnel: w1174 -> [w1245]
                      i -> [w1256]
                      stop <- w1259 stop-if-true
                      (unwired) FALSE ("Log (T)")
                      n280 = Index Array(array=w1262, index=w1256) -> ()  [unwired: 1 out]
                      n281 = Index Array(array=w1257, index=w1256) -> (element=w1248:string)
                      n282 = call <vilib>:"Space Constant.vi"() -> ("String"=w1246:string)
                      n283 = Concatenate Strings(w1248, w1246, w1245) -> (w1247:string)
                      n284 = call "Delay T4.vi"("milliseconds to wait"=u32 10, "error in (no error)"=w1244) -> ("error out"=w1252:errorcluster)  [unwired: 9 in]
                      n285 = local write "STATUS"(w1247) -> ()
                      n286 = call "WS1050 AD7747 READ 36 DUT.vi"("error in"=w1252, "Log (T)"=FALSE, "DUT Mask Mode (All)"=WSVCAP_SHL_I2C_DUT_Mask_Mode_Enum."C1") -> ("error out"=w1254:errorcluster, "AD7747 Values"=w1253:string[][])  [unwired: 7 in]
                      n287 = for {
                        tunnel: [w1265] -> w1258 mode=indexing
                        tunnel: w1254 -> [w1264]
                        tunnel: [w1264] -> w1250
                        tunnel: w1253 -> [w1263] mode=indexing
                        n288 = Index Array(array=w1263, index=1) -> (element=w1265:string)
                      }
                      n289 = Unbundle By Name(w1250) -> ("status"=w1261:bool)
                      n290 = Or(x=w1261, y=w1260) -> (x .or. y?=w1259:bool)
                    }
                    n291 = Transpose 2D Array(2D array=w1187) -> (transposed array=w1177:string[][])
                    "VPI C1" <- w1177
                    n292 = Array Size(array=w1193) -> (size(s)=w1186:i32)
                    n293 = for {
                      N: w1186 -> [_]
                      tunnel: w1192 -> [w1239]
                      tunnel: w1185 -> [w1237]
                      tunnel: [w1236] -> w1181
                      tunnel: [w1235] -> w1184 mode=indexing
                      tunnel: w1193 -> [w1234]
                      tunnel: w1180 -> [w1221]
                      tunnel: [w1227] -> w1179
                      tunnel: w1174 -> [w1223]
                      i -> [w1233]
                      stop <- w1236 stop-if-true
                      (unwired) FALSE ("Log (T)")
                      n294 = Index Array(array=w1239, index=w1233) -> ()  [unwired: 1 out]
                      n295 = Index Array(array=w1234, index=w1233) -> (element=w1225:string)
                      n296 = call <vilib>:"Space Constant.vi"() -> ("String"=w1224:string)
                      n297 = Concatenate Strings(w1225, w1224, w1223) -> (w1222:string)
                      n298 = call "Delay T4.vi"("milliseconds to wait"=u32 10, "error in (no error)"=w1221) -> ("error out"=w1229:errorcluster)  [unwired: 9 in]
                      n299 = call "WS1050 AD7747 READ 36 DUT.vi"("error in"=w1229, "Log (T)"=FALSE, "DUT Mask Mode (All)"=WSVCAP_SHL_I2C_DUT_Mask_Mode_Enum."C2") -> ("error out"=w1231:errorcluster, "AD7747 Values"=w1230:string[][])  [unwired: 7 in]
                      n300 = local write "STATUS"(w1222) -> ()
                      n301 = for {
                        tunnel: [w1242] -> w1235 mode=indexing
                        tunnel: w1231 -> [w1241]
                        tunnel: [w1241] -> w1227
                        tunnel: w1230 -> [w1240] mode=indexing
                        n302 = Index Array(array=w1240, index=3) -> (element=w1242:string)
                      }
                      n303 = Unbundle By Name(w1227) -> ("status"=w1238:bool)
                      n304 = Or(x=w1238, y=w1237) -> (x .or. y?=w1236:bool)
                    }
                    n305 = Transpose 2D Array(2D array=w1184) -> (transposed array=w1176:string[][])
                    "VPI C2" <- w1176
                    n306 = Array Size(array=w1191) -> (size(s)=w1183:i32)
                    n307 = for {
                      N: w1183 -> [_]
                      tunnel: w1190 -> [w1216]
                      tunnel: w1181 -> [w1214]
                      tunnel: [w1213] -> w1189
                      tunnel: [w1212] -> w1182 mode=indexing
                      tunnel: w1191 -> [w1211]
                      tunnel: w1179 -> [w1198]
                      tunnel: [w1204] -> w1188
                      tunnel: w1174 -> [w1200]
                      i -> [w1210]
                      stop <- w1213 stop-if-true
                      (unwired) FALSE ("Log (T)")
                      n308 = Index Array(array=w1216, index=w1210) -> ()  [unwired: 1 out]
                      n309 = Index Array(array=w1211, index=w1210) -> (element=w1202:string)
                      n310 = call <vilib>:"Space Constant.vi"() -> ("String"=w1199:string)
                      n311 = call "Delay T4.vi"("milliseconds to wait"=u32 10, "error in (no error)"=w1198) -> ("error out"=w1206:errorcluster)  [unwired: 9 in]
                      n312 = Concatenate Strings(w1202, w1199, w1200) -> (w1201:string)
                      n313 = call "WS1050 AD7747 READ 36 DUT.vi"("error in"=w1206, "Log (T)"=FALSE, "DUT Mask Mode (All)"=WSVCAP_SHL_I2C_DUT_Mask_Mode_Enum."C3") -> ("error out"=w1208:errorcluster, "AD7747 Values"=w1207:string[][])  [unwired: 7 in]
                      n314 = local write "STATUS"(w1201) -> ()
                      n315 = for {
                        tunnel: [w1219] -> w1212 mode=indexing
                        tunnel: w1208 -> [w1218]
                        tunnel: [w1218] -> w1204
                        tunnel: w1207 -> [w1217] mode=indexing
                        n316 = Index Array(array=w1217, index=5) -> (element=w1219:string)
                      }
                      n317 = Unbundle By Name(w1204) -> ("status"=w1215:bool)
                      n318 = Or(x=w1215, y=w1214) -> (x .or. y?=w1213:bool)
                    }
                    n319 = Transpose 2D Array(2D array=w1182) -> (transposed array=w1175:string[][])
                    "VPI C3" <- w1175
                  }
                }
                n320 = call "Delay T4.vi"("milliseconds to wait"=u32 10, "error in (no error)"=w1098) -> ("error out"=w1118:errorcluster)  [unwired: 9 in]
              }
              frame #5 {
                n321 = case shown="False" w1267 {
                  tunnel: w1304 -> [w1318 w1320]
                  tunnel: [w1318 w1319] -> w1278
                  tunnel: [w1317 w1326] -> w1294
                  tunnel: w1295 -> [w1317 w1325]
                  tunnel: [w1315 w1323] -> w1283
                  tunnel: [w1315 w1322] -> w1280
                  tunnel: [w1315 w1321] -> w1277
                  tunnel: [string[][] [] w1324] -> w1284
                  frame False {
                    w1315 = string[][] []
                  }
                  frame True {
                    n322 = for {
                      tunnel: "VSA Voltage(V)" -> [w1350] mode=indexing
                      tunnel: [w1354] -> w1326
                      tunnel: w1325 -> [w1352]
                      tunnel: [w1351] -> w1323 mode=indexing
                      tunnel: [w1338] -> w1322 mode=indexing
                      tunnel: [w1347] -> w1324 mode=indexing
                      tunnel: [w1332] -> w1321 mode=indexing
                      tunnel: w1320 -> [w1331]
                      tunnel: [w1330] -> w1319
                      w1329 = FALSE ("Log (T)")
                      w1346 = u16 0 items=["Voltage", "Current"] ("Source Mode  (0: Voltage)")
                      n323 = call "Configure Output.vi"("Source Mode  (0: Voltage)"=w1346, "error in (no error)"=w1331, "Compliance  Level (0.1)"=0.1, "Output Level (0)"=w1350, "VISA resource name"=w1352) -> ("error out"=w1358:errorcluster, "VISA resource name out"=w1356:refnum<visa-resource-name>)  [unwired: 5 in]
                      n324 = Number To Fractional String(number=w1350) -> (F-format string=w1349:string)  [unwired: 3 in]
                      n325 = call "Enable Output.vi"("error in (no error)"=w1358, "Enable Output (T: Enable)"=TRUE, "VISA resource name"=w1356) -> ("error out"=w1359:errorcluster, "VISA resource name out"=w1354:refnum<visa-resource-name>)  [unwired: 7 in]
                      n326 = call "Delay T4.vi"("milliseconds to wait"=u32 10, "error in (no error)"=w1359) -> ("error out"=w1345:errorcluster)  [unwired: 9 in]
                      n327 = call "WS1050 AD7747 READ 36 DUT.vi"("error in"=w1345, "Log (T)"=w1329, "DUT Mask Mode (All)"=WSVCAP_SHL_I2C_DUT_Mask_Mode_Enum."C1") -> ("error out"=w1342:errorcluster, "AD7747 Values"=w1344:string[][])  [unwired: 7 in]
                      n328 = for {
                        tunnel: w1344 -> [w1370] mode=indexing
                        tunnel: [w1371] -> w1351 mode=indexing
                        tunnel: w1342 -> [w1369]
                        tunnel: [w1369] -> w1341
                        n329 = Index Array(array=w1370, index=1) -> (element=w1371:string)
                      }
                      n330 = for {
                        N: 36 -> [_]
                        tunnel: w1349 -> [w1368]
                        tunnel: [w1368] -> w1347 mode=indexing
                      }
                      n331 = call "WS1050 AD7747 READ 36 DUT.vi"("error in"=w1341, "Log (T)"=w1329, "DUT Mask Mode (All)"=WSVCAP_SHL_I2C_DUT_Mask_Mode_Enum."C2") -> ("error out"=w1339:errorcluster, "AD7747 Values"=w1337:string[][])  [unwired: 7 in]
                      n332 = for {
                        tunnel: w1337 -> [w1365] mode=indexing
                        tunnel: [w1366] -> w1338 mode=indexing
                        tunnel: w1339 -> [w1364]
                        tunnel: [w1364] -> w1336
                        n333 = Index Array(array=w1365, index=3) -> (element=w1366:string)
                      }
                      n334 = call "WS1050 AD7747 READ 36 DUT.vi"("error in"=w1336, "Log (T)"=w1329, "DUT Mask Mode (All)"=WSVCAP_SHL_I2C_DUT_Mask_Mode_Enum."C3") -> ("error out"=w1334:errorcluster, "AD7747 Values"=w1333:string[][])  [unwired: 7 in]
                      n335 = for {
                        tunnel: w1333 -> [w1361] mode=indexing
                        tunnel: [w1362] -> w1332 mode=indexing
                        tunnel: w1334 -> [w1360]
                        tunnel: [w1360] -> w1330
                        n336 = Index Array(array=w1361, index=5) -> (element=w1362:string)
                      }
                    }
                    n337 = local write "STATUS"("VSA Testing...." ("STATUS")) -> ()
                  }
                }
                n338 = Transpose 2D Array(2D array=w1284) -> (transposed array=w1282:string[][])
                n339 = Transpose 2D Array(2D array=w1283) -> (transposed array=w1281:string[][])
                n340 = Transpose 2D Array(2D array=w1280) -> (transposed array=w1279:string[][])
                n341 = Transpose 2D Array(2D array=w1277) -> (transposed array=w1276:string[][])
                n342 = call "WS1050_VSA_Convert_Data.vi"("VSA_C3"=w1276, "error in (no error)"=w1278, "VSA_C2"=w1279, "VSA_C1"=w1281, "Voltage"=w1282) -> ("error out"=w1275:errorcluster, "VSA_V3"=w1272:string[][], "VSA_V2"=w1273:string[][], "VSA_V1"=w1274:string[][])  [unwired: 3 in]
                "VSA_V1" <- w1274
                "VSA_V2" <- w1273
                "VSA_V3" <- w1272
                n343 = case shown="True" w1267 {
                  tunnel: w1294 -> [w1308 w1314]
                  tunnel: [w1308 w1313] -> w1293
                  tunnel: w1275 -> [w1307 w1312]
                  tunnel: [w1307 w1309] -> w1292
                  frame False {
                  }
                  frame True {
                    w1310 = u16 0 items=["Voltage", "Current"] ("Source Mode  (0: Voltage)")
                    n344 = call "Configure Output.vi"("Source Mode  (0: Voltage)"=w1310, "error in (no error)"=w1312, "Output Level (0)"=0.0, "VISA resource name"=w1314) -> ("error out"=w1309:errorcluster, "VISA resource name out"=w1313:refnum<visa-resource-name>)  [unwired: 6 in]
                  }
                }
                n345 = call "Delay T4.vi"("milliseconds to wait"=u32 50, "error in (no error)"=w1292) -> ("error out"=w1291:errorcluster)  [unwired: 9 in]
              }
              frame #6 {
                # "Handshake Check and EFuse Readback"
                n346 = Or(x=w1382, y=w1387) -> (x .or. y?=w1373:bool)
                n347 = case shown="True" w1373 {
                  tunnel: w1409 -> [w1422 _]
                  tunnel: w1408 -> [w1421 w1427]
                  tunnel: [w1420 w1427] -> w1407
                  tunnel: w1406 -> [w1419 _]
                  tunnel: w1405 -> [w1418 _]
                  tunnel: w1404 -> [w1417 _]
                  tunnel: [w1413 w1426] -> w1403
                  tunnel: [w1412 w1426] -> w1398
                  tunnel: w1374 -> [w1411 _]
                  tunnel: w1392 -> [w1410 _]
                  frame False {
                    n348 = call "WS1050_36DUT_Handshake Check R1_Record All Regs Ver1.0.vi"("file path (use dialog)"=w1422, "Reg1_Bit Cntrl"="Reg1_Bit Cntrl", "File Name"=w1410, "SN"=w1417, "Loop"=w1411, "error"=w1421, "Lot #"=w1419, "Wafer #"=w1418) -> ("Pass/Fail"=→"EFuse Readback Status":bool[], "EFuse Read back"=w1412:string[], "Status"=w1413:string[], "error out"=w1420:errorcluster)  [unwired: 6 in, 2 out]
                    n349 = case shown="0" w1411 {
                      tunnel: w1412 -> [w1423 w1424]
                      frame 0 {
                        "EFuse RB T0" <- w1423
                      }
                      frame 1, Default {
                        "Current EFuse Read back" <- w1424
                      }
                    }
                    n350 = local write "STATUS"("Hand Shake & EFuse Readback...." ("STATUS")) -> ()
                  }
                  frame True {
                    n351 = for {
                      N: 36 -> [_]
                      tunnel: ["NA"] -> w1426 mode=indexing
                    }
                  }
                }
                n352 = Build Array(w1396, w1394, w1393) -> (w1395:string[])
              }
              frame #7 {
                # "Save Data"
                n353 = Increment(x=w1440) -> (x+1=w1439:i32)
                n354 = local write "STATUS"("Saving Data...." ("STATUS")) -> ()
                n355 = Multiply(x=w1439, y=36) -> (x*y=w1434:i32)
                n356 = Path To String(path=w1444) -> (string=w1443:string)
                n357 = Bundle("Test Program"=w1470, "Comment"=w1469, "Data Out"=w1450, "Data Out"=w1449, "Data Out"=w1429, w1448, "Data Out"=w1447, "Data Out"=w1446, "Data Out"=w1445, "Freq(Hz)"=w1432, "Board#"=w1430) -> (w1431:T8)  [unwired: 1 in]
                n358 = case shown="True" "Debug" {
                  tunnel: w1434 -> [w1477 w1480]
                  tunnel: [w1477 w1478] -> w1433
                  frame False {
                  }
                  frame True {
                    n359 = Multiply(x=w1480, y="No of Rows\nFrom Spread Sheet") -> (x*y=w1478:i32)
                  }
                }
                n360 = call "WS1050_36 DUT CV Curve SData Ver1.0.vi"("TMN DC\\CAP Data Log File Path"=w1444, "Lot#"=w1472, "VSA_V1"=w1458, "Wafer#"=w1468, "File Name"=w1437, "error in"=w1475, "TP/Comment"=w1431, "EFuse"=w1462, "Data Output C3"=w1452, "Temperature"=w1456, "VSA_V2"=w1459, "VPI C3"=w1454, "Data Output C1"=w1465, "VPI C2"=w1453, "SN"=w1473, "R/W Status"=w1471, "Cap Header"=w1455, "HD/Cycles Completed"=w1461, "Data Output C2"=w1451, "VSA_V3"=w1457, "Current"=w1464, "VPI C1"=w1463) -> ("error out"=w1474:errorcluster)  [unwired: 5 in]
                n361 = Concatenate Strings(w1443, "\\" ("string"), w1437, "_Multi Socket Data.csv" ("string")) -> (w1442:string)
              }
              frame #8 {
                n362 = case shown="True" "Plot Delta Cmin" {
                  tunnel: w1488 -> [w1504 w1522]
                  tunnel: [w1504 w1518] -> w1482
                  tunnel: w1487 -> [_ w1514]
                  tunnel: w1485 -> [_ w1508]
                  frame False {
                  }
                  frame True {
                    n363 = String To Path(string=w1514) -> (path=w1513:path)
                    n364 = call "Delay T4.vi"("milliseconds to wait"=u32 50, "error in (no error)"=w1522) -> ("error out"=w1521:errorcluster)  [unwired: 9 in]
                    n365 = call "36DUT Plot From Spread Sheet Updated.vi"("Col C2"="Col C2", "Col C3"="Col C3", "Plot"="Plot", "No of Rows"=w1508, "error in (no error)"=w1521, "Col C1"="Col C1", "Bank"="Bank 1", "file path (dialog if empty)"=w1513) -> ("error out"=w1516:errorcluster, "Delta C_Min Plot"=→"DeltaC Change_1":dbl[][])  [unwired: 2 in]
                    n366 = call "36DUT Plot From Spread Sheet Updated.vi"("Col C2"="Col C2", "Col C3"="Col C3", "Plot"="Plot", "No of Rows"=w1508, "error in (no error)"=w1516, "Col C1"="Col C1", "Bank"="Bank 2", "file path (dialog if empty)"=w1513) -> ("error out"=w1517:errorcluster, "Delta C_Min Plot"=→"DeltaC Change_2":dbl[][])  [unwired: 2 in]
                    n367 = call "36DUT Plot From Spread Sheet Updated.vi"("Col C2"="Col C2", "Col C3"="Col C3", "Plot"="Plot", "No of Rows"=w1508, "error in (no error)"=w1517, "Col C1"="Col C1", "Bank"="Bank 3", "file path (dialog if empty)"=w1513) -> ("error out"=w1518:errorcluster, "Delta C_Min Plot"=→"DeltaC Change_3":dbl[][])  [unwired: 2 in]
                  }
                }
                n368 = Get Date/Time In Seconds() -> (seconds since 1Jan1904=w1491:timestamp)
                n369 = Get Date/Time String(seconds (now)=w1491, want seconds? (F)=TRUE) -> (date string=→"date string":string, time string=→"Previous Time":string)  [unwired: 1 in]
                n370 = Greater Or Equal?(x=w1484, y="TTF Completed") -> (x >= y?=w1483:bool)
                n371 = case shown="True" w1483 {
                  tunnel: w1482 -> [w1497 w1499]
                  tunnel: [w1497 w1498] -> w1481
                  frame False {
                  }
                  frame True {
                    n372 = call "Delay T4.vi"("milliseconds to wait"=u32 50, "error in (no error)"=w1499) -> ("error out"=w1502:errorcluster)  [unwired: 9 in]
                    n373 = call "WSVCAP SHL Host TL RFFE Write - Multiple DUTs - Common Data.vi"("Data Out"="070201000000", "error in"=w1502, "Log (T)"=FALSE) -> ("error out"=w1498:errorcluster)  [unwired: 12 in]
                  }
                }
                "Loop Completed" <- w1484
              }
            }
            n374 = Compound Arithmetic op=OR(w523, w546) -> (w552:bool)
            n375 = call "Delay T4.vi"("milliseconds to wait"=u32 10, "error in (no error)"=w454) -> ("error out"=w455:errorcluster)  [unwired: 9 in]
          }
          n376 = Unbundle By Name(w389) -> ("status"=w396:bool)
          n377 = Compound Arithmetic op=OR(w396, w395, w394) -> (w385:bool)
        }
        n378 = for {
          tunnel: w275 -> [w1534]
          tunnel: w255 -> [w1533]
          tunnel: w301 -> [w1531] mode=indexing
          tunnel: [w1526] -> w273
          tunnel: [w1530] -> w300
          n379 = call "E3631A_Voltage Controller.vi"("VISA resource name"=w1533, "I_VDD(A)"=0.5, "Channel Controller"=w1531, "Voltage 1"=0.0, "Voltage 2"=3.3, "error in (no error)"=w1534, "I_3.3V (A)"=0.5) -> ("VISA resource name out"=w1530:refnum<visa-resource-name>, "error out"=w1527:errorcluster)  [unwired: 7 in]
          n380 = call "Delay T4.vi"("milliseconds to wait"=u32 100, "error in (no error)"=w1527) -> ("error out"=w1526:errorcluster)  [unwired: 9 in]
        }
        n381 = VISA Write(VISA resource name=w291, write buffer="SOUR:FUNC VOLT;VOLT:MODE FIX;RANG 100;LEV 0.0;:SENS:FUNC \"CURR\";CURR:PROT 60E-3;RANG 100E-3;:OUTP ON", error in (no error)=w275) -> (VISA resource name out=w289:refnum<visa-resource-name>, error out=w274:errorcluster)  [unwired: 1 out]
        n382 = Merge Errors(w273, w274) -> (w290:errorcluster)
      }
      frame True {
      }
    }
    n383 = Wait Until Next ms Multiple(millisecond multiple=u32 100) -> ()  [unwired: 1 out]
    n384 = Unbundle By Name(w64) -> ("status"=w81:bool)
    n385 = Or(x=w81, y=w73) -> (x .or. y?=w80:bool)
    "STATUS" <- "Idle...." ("STATUS")
  }
  "Ke2000 Out" <- w21
  "PS1 Out" <- w20
  n386 = local write "stop"(w7) -> ()
  n387 = case shown="True" w18 {
    tunnel: [w1551 w1554] -> w2
    tunnel: w12 -> [w1551 w1553]
    frame False {
    }
    frame True {
      n388 = local write "Online"(FALSE ("Online")) -> ()
      n389 = call "WSVCAP SHL Host TL Close.vi"("error in"=w1553) -> ("error out"=w1554:errorcluster)  [unwired: 14 in]
    }
  }
  "error out" <- w2
  n390 = VISA Write(VISA resource name=w13, write buffer="SOUR:FUNC VOLT;VOLT:MODE FIX;RANG 100;LEV 0.0;:SENS:FUNC \"CURR\";CURR:PROT 60E-3;RANG 100E-3;:OUTP OFF", error in (no error)=w12) -> (VISA resource name out=→"VISA resource name out":refnum<visa-resource-name>, error out=→"error out 2":errorcluster)  [unwired: 1 out]
